vi "SpectrometerSpinCoater_v08.vi"() -> ()   [LabVIEW 2018]
uses:
  <instrlib>/Classes/CCD/Abstract_CCD/Abstract_CCD.lvclass
  <instrlib>/Classes/SpinCoater/SpinCoater.lvclass
  TypDef/DeviceQueue_TypeDef.ctl
  TypDef/DeviceQueue_Action.ctl
  TypDef/TabControl.ctl
  TypDef/DataQueue_TypeDef.ctl
  TypDef/DataQueue_Action.ctl
  <vilib>/Utility/error.llb/DialogType.ctl
  <instrlib>/Classes/CCD/Avantes/Avantes.lvclass
  C:/Program Files/National Instruments/LabVIEW 2018/instr.lib/Classes/CCD/Abstract_CCD/Abstract_CCD.lvclass
  <vilib>/Analysis/baseanly.llb/A x Vector.vi
  <vilib>/Analysis/NI_AALBase.lvlib
panel:
  out "Nr After Spin":u16=6
  out "Action":string="TimeOut"
  out "Time.spin":refnum<file>
  out "Meas.spin":refnum<file>
  out "Arduino":bool
  out "NKT":bool
  out "Spectromter":bool
  in  "Abort Button":bool
  in  "Stop Button":bool=TRUE
  in  "Tab Control":T1(tab)
  in  "Spin at end":bool=TRUE
  in  "Duration after":dbl[unit]=10.0
  in  "periodic time":dbl[unit]=2.0
  in  "Program Spin Coater":T2(array[cluster])=[{"Speed (rpm)"=1500.0, "Time (s)"=5.0, "Acc (rpm/s)"=0.0}]
  in  "Spectra Count":u16
  in  "Measure_MeasureSpectrum":bool
  out "Overall Time":dbl=6.5
  in  "Seconds after Spin":dbl[unit]=0.5
  in  "Seconds to Spin":dbl[unit]=1.0
  in  "Calculate Frames":bool=TRUE
  in  "Frames":i32=17106
  in  "StartMeasurement_Button":bool
  in  "Measure_Preview":bool
  out "Measure_Graph":T3(graph) caption="XY Graph"
  in  "Measure_FramesSpectrometer":dbl=200.0 caption="Frames for Spectrometer"
  in  "StartSpin_Button":bool
  in  "Record RefSpec":bool
  in  "Record_Darkspec":bool
  in  "Measure_Comments":string="Just for testing" caption="Comments"
  in  "Measure_FileName":string="TestingAfter" caption="File Name"
  in  "Measure_SavePath":path=path "C:/Users/Timo/Desktop/Test/180824" caption="Save Path"
  out "Measure_FrameRate":dbl[unit]=2631.5791015625 caption="Frame Rate"
  in  "Measure_IntegrationTime":dbl[unit]=3e-05 caption="Integration Time"
  in  "Dividider Get Spectra":u32=1 min=1
  in  "Automatically \nadjust count":bool=TRUE
  in  "Reset Count\nafter Spin Coating":bool=TRUE
  in  "Speed":dbl
  in  "Milliseconds":dbl
  in  "Debug":bool
  in  "Port Arduino":refnum<visa-resource-name>="COM3"
  out "Error Arduino":bool caption="Error"
  in  "Init_Arduino":bool=TRUE caption="Init"
  out "Caption_Settings_Arduino":string="Arduino"
  out "Caption_Settings_NKT":string="NKT Laser"
  out "Error_Spectromter":bool caption="Error"
  in  "Init_Spectrometer":bool=TRUE caption="Init"
  out "Caption_Settings_Spectrometer":string="Spectromter"
  # "Speed (rpm)   Time (s)        Acceleration \n                                               (rpm/s)"
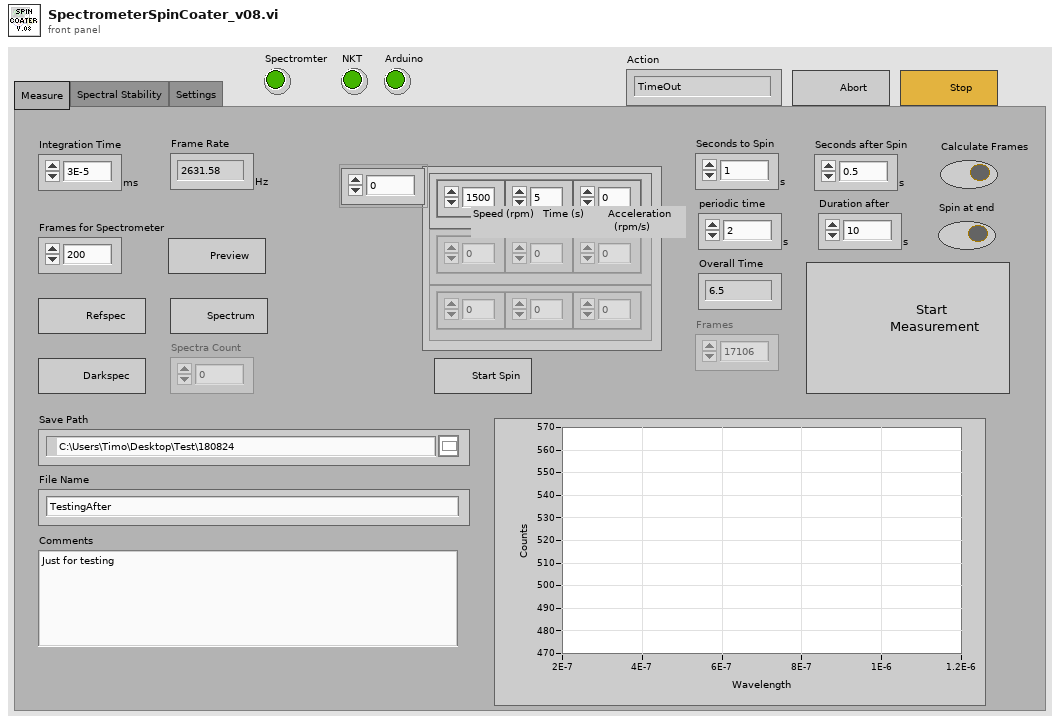
[diagram p1: front panel]
types:
  T1 = enum32{"Measure", "Spectral Stability", "Settings"}
  T2 = cluster{"Speed (rpm)":dbl, "Time (s)":dbl, "Acc (rpm/s)":dbl}[]
  T3 = cluster{"Wavlength":dbl[unit][], "Image":dbl[]}[]
  T4 = cluster{"Dark":cluster{"Image":dbl[][][], "Frame Size":cluster{"F":i32, "Y":i32, "X":i32}}[], "Ref":cluster{"Image":dbl[][][], "Frame Size":cluster{"F":i32, "Y":i32, "X":i32}}[], "Wavlength":dbl[unit][], "spec":dbl[][]}
  T5 = cluster{"Abstract_CCD.lvclass":refnum<class "Abstract_CCD.lvclass">, "SpinCoater.lvclass":refnum<class "SpinCoater.lvclass">}
  T6 = typedef "DataQueue_TypeDef.ctl" = cluster{"QueueAction":T7, "Data":cluster{"Image":dbl[][][], "Frame Size":cluster{"F":i32, "Y":i32, "X":i32}}[], "Data_Raw":cluster{"Image":dbl[][][], "Frame Size":cluster{"F":i32, "Y":i32, "X":i32}}[], "Data_Dark":cluster{"Image":dbl[][][], "Frame Size":cluster{"F":i32, "Y":i32, "X":i32}}[], "Data_Ref":cluster{"Image":dbl[][][], "Frame Size":cluster{"F":i32, "Y":i32, "X":i32}}[], "Device Information":string[], "Numeric Control":dbl, "Boolean":bool, "Wavelength":dbl[unit][], "Time":dbl[], "Time Stamp":timestamp, "Numeric Control 2":dbl, "TabControl":T8}
  T7 = typedef "DataQueue_Action.ctl" = enum16{"TimeOut", "Close_Program", "Stop_Measurement", "Measure_InSituSpinCoating", "Measure_Spectrum", "Measure_SpectrumAdvanced", "Save_InSitu", "Save_SpectralStability", "Set_Ref", "Set_Dark", "Set_Wavelength", "Spectrometer_Measure", "Spectrometer_Preview", "Transfer_Settings"}
  T8 = typedef "TabControl.ctl" = enum16{"Measure", "Spectral Stability", "Settings"}
  T9 = typedef "DeviceQueue_TypeDef.ctl" = cluster{"QueueAction":T10, "Numeric 1":dbl, "Numeric 2":dbl, "Boolean 1":bool, "Boolean 2":bool, "Spin Program":dbl[][], "Spin Prg v07":cluster{"Speed (rpm)":dbl, "Time (s)":dbl, "Acc (rpm/s)":dbl}[], "Time Stamp":timestamp, "TabControl":T8}
  T10 = typedef "DeviceQueue_Action.ctl" = enum16{"TimeOut", "Wait", "Close_Program", "Abort", "Spectrometer_Init", "Spectrometer_Close", "Spectrometer_DeviceInformation", "Spectrometer_Measure", "Spectrometer_MeasureAdvanced", "Spectrometer_Preview", "Spectrometer_Abort", "Spectrometer_StartMeasurement", "Spectrometer_GetData", "Spectrometer_StopMeasurement", "Spectrometer_SetIntegrationTime", "Spectrometer_SetFrames", "Spectrometer_SetDarkspec", "Spectrometer_SetReference", "Spectrometer_SetTriggerMode", "Laser_Init", "Laser_Close", "Arduino_Init", "Arduino_Close", "Arduino_LoadProgram", "Arduino_StartProgram", "Arduino_SetSpeed", "Arduino_SetMillis", "Arduino_StopSpin", "Measure_InSitu", "Measure_Spectrum", "Measure_InSituAdvanced", "Measure_Stop"}
  T11 = enum16{"open", "replace", "create", "open or create", "replace or create", "replace or create with confirmation"}
  T12 = cluster{"Image":dbl[][][], "Frame Size":cluster{"F":i32, "Y":i32, "X":i32}}[]
  T13 = cluster{"Image":dbl[][][], "Frame Size":cluster{"F":i32, "Y":i32, "X":i32}}
  T14 = cluster{"Wavlength":dbl[unit][], "A x Vector":dbl[]}
  T15 = cluster{"Wavlength":dbl[unit][], "A x Vector":dbl[]}[]
  T16 = cluster{u16[][], u16[][], dbl[], "Numeric Control":dbl, "Numeric Control 2":dbl}
  T17 = typedef "DialogType.ctl" = u16
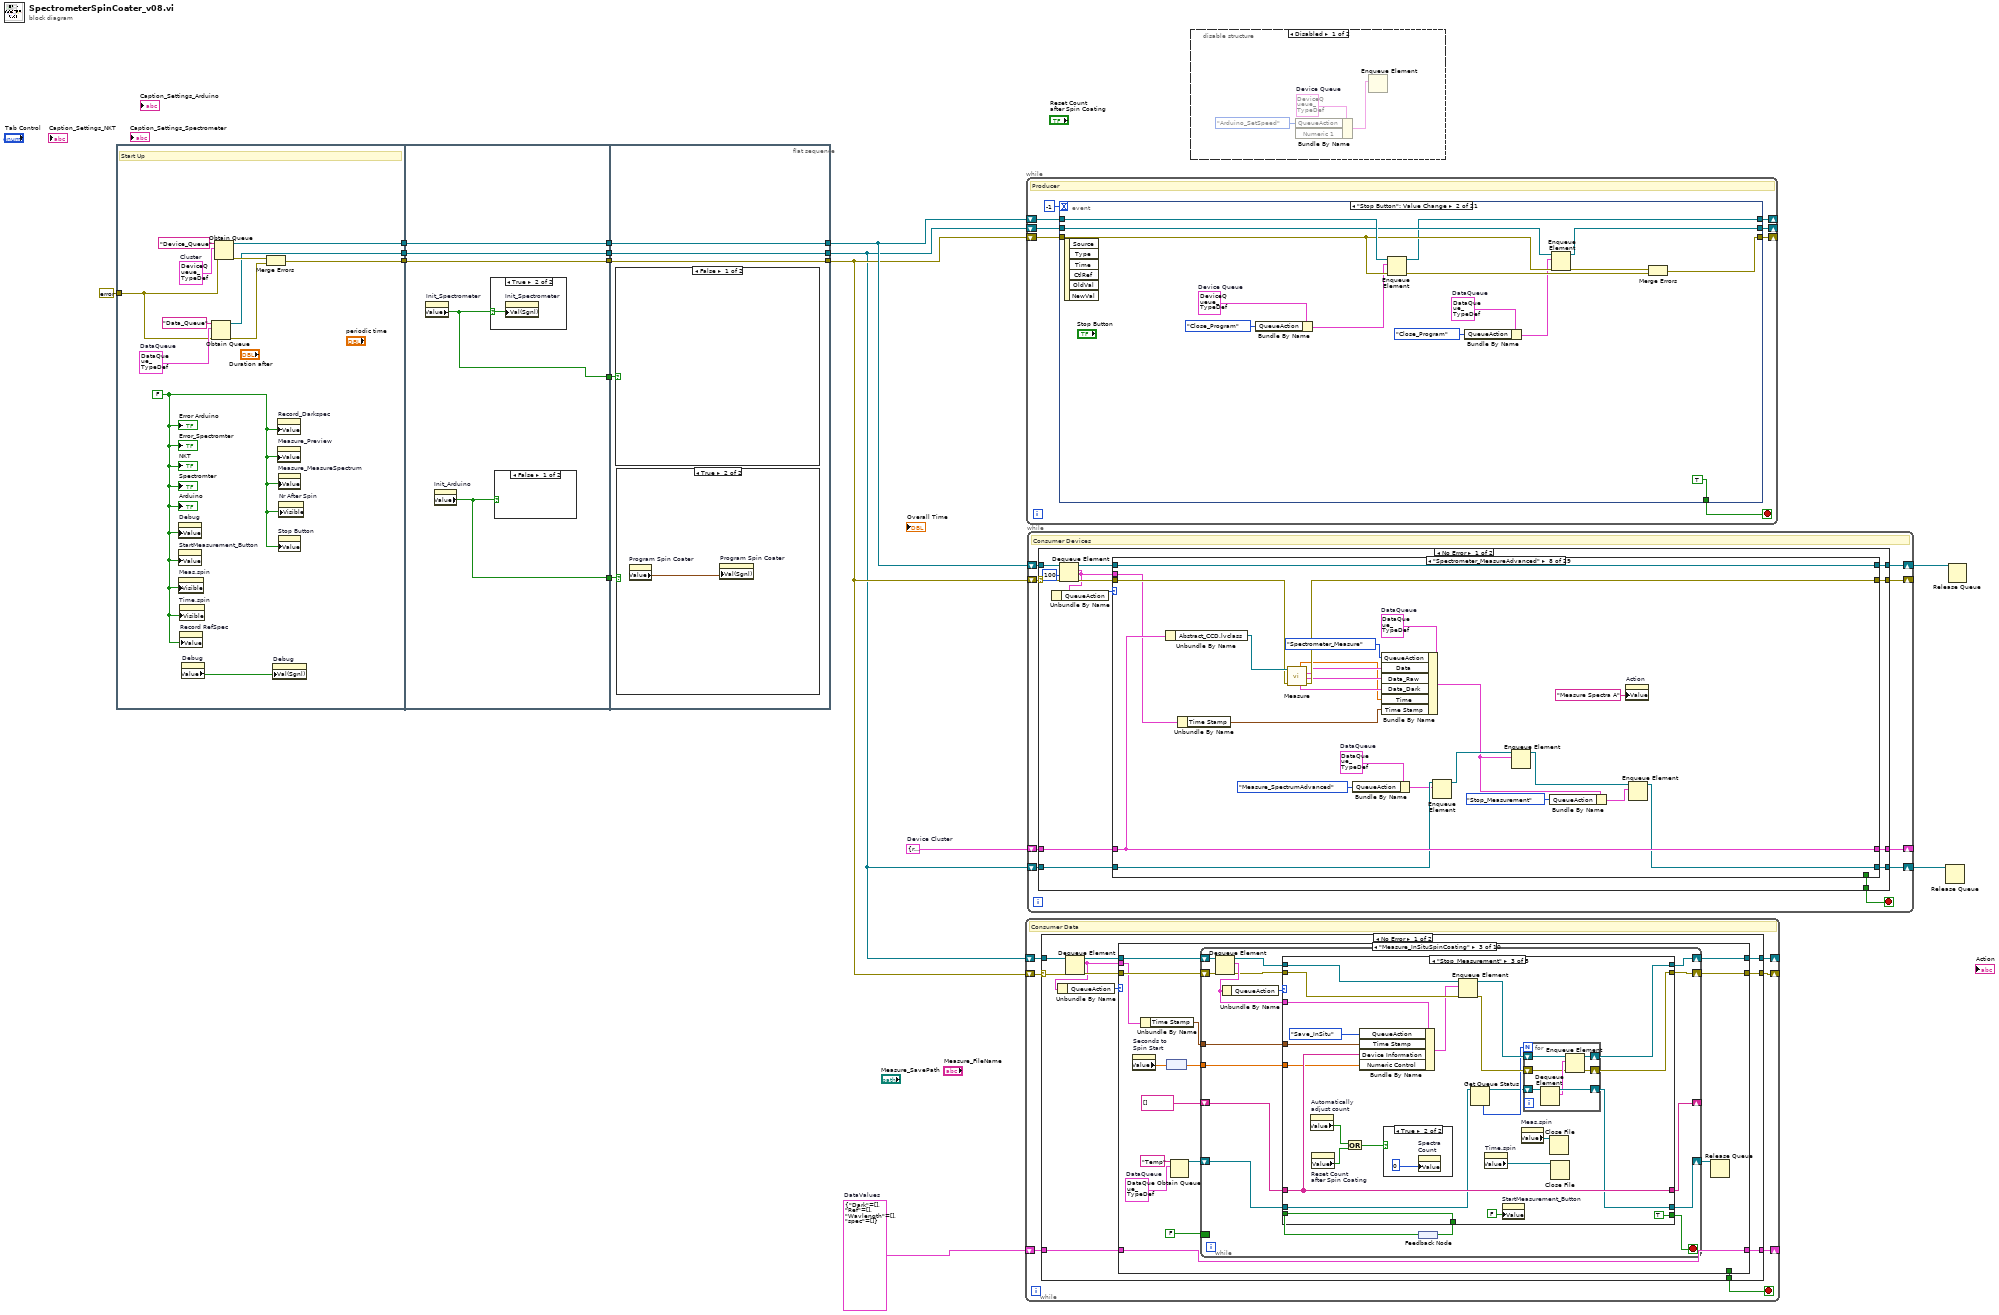
[diagram p0: block diagram]
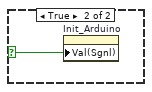
[diagram p3: hidden frame]
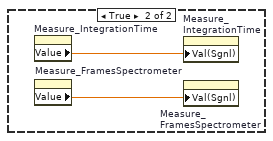
[diagram p6: hidden frame]
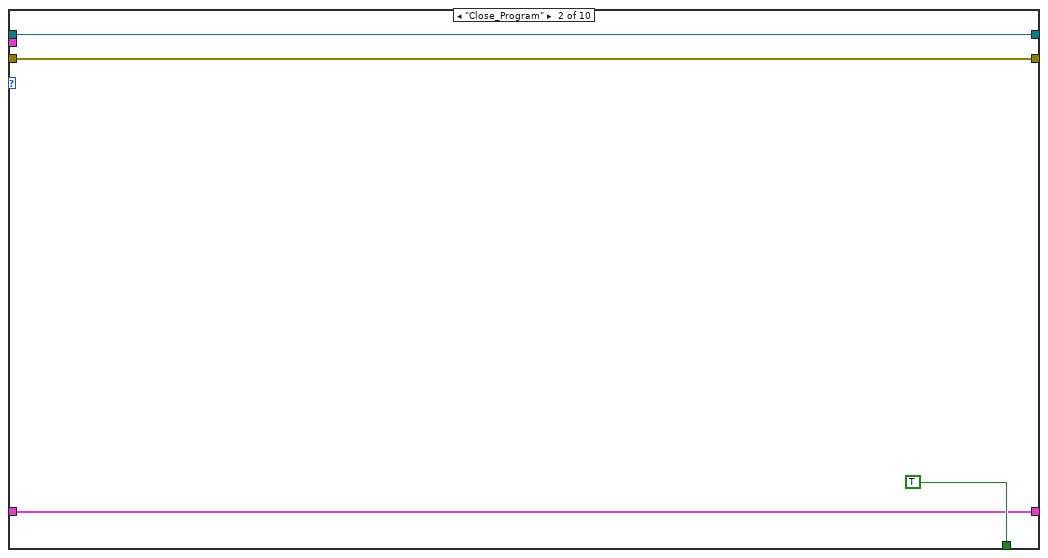
[diagram p8: hidden frame]
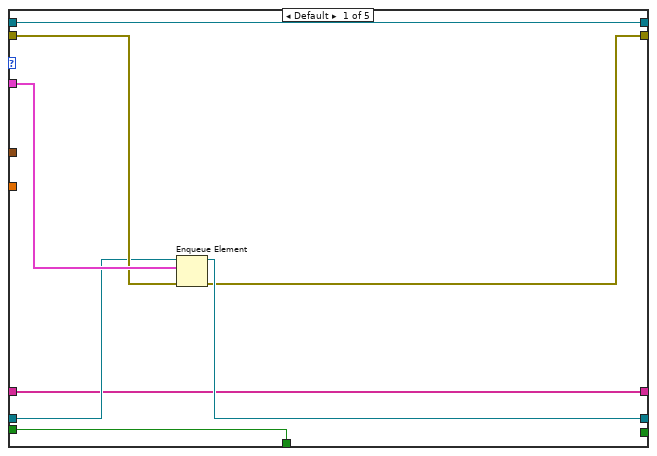
[diagram p9: hidden frame]
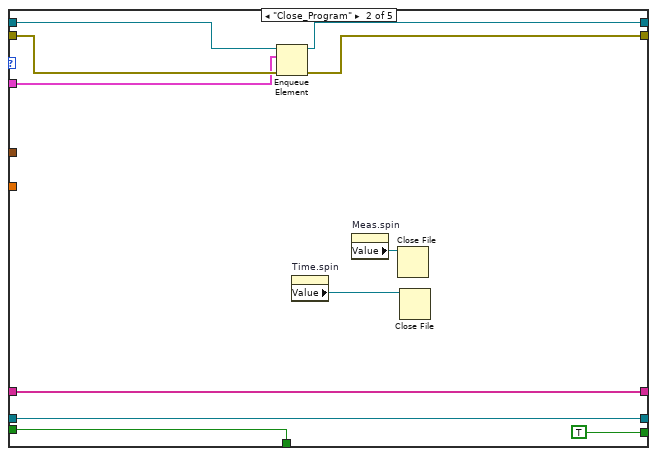
[diagram p10: hidden frame]
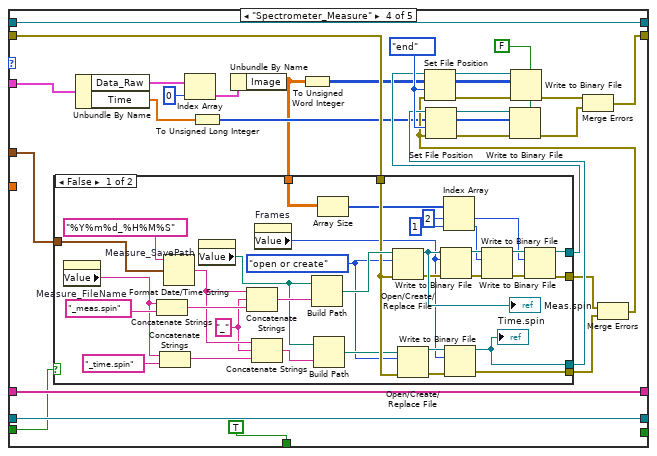
[diagram p12: hidden frame]
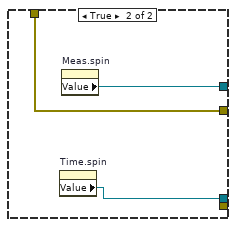
[diagram p13: hidden frame]
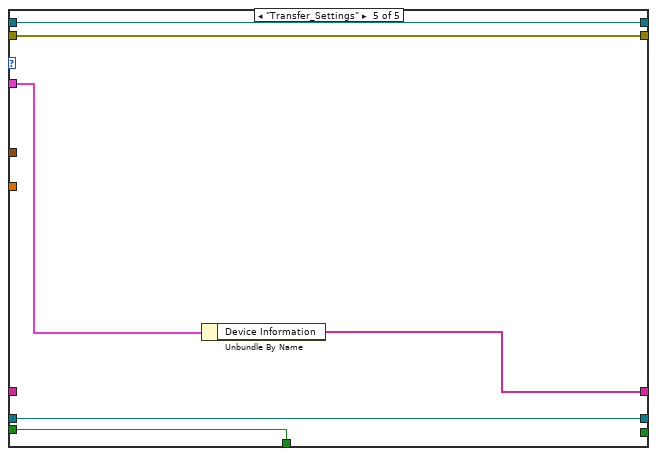
[diagram p14: hidden frame]
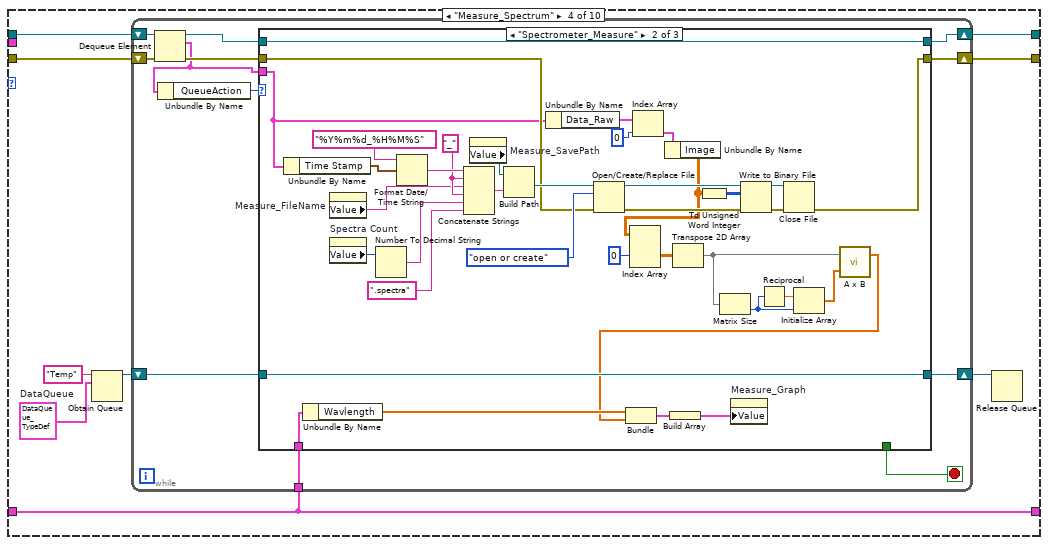
[diagram p15: hidden frame]
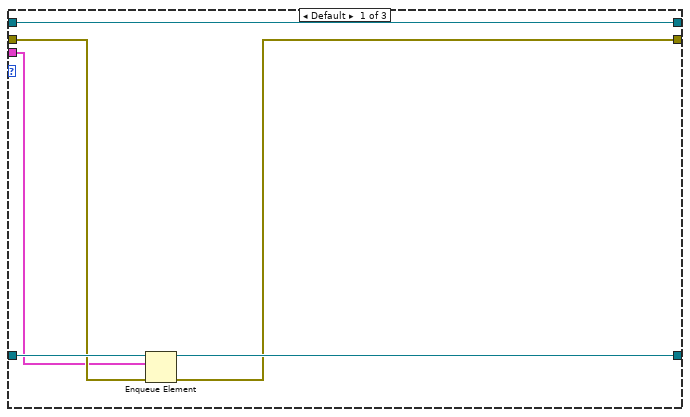
[diagram p16: hidden frame]
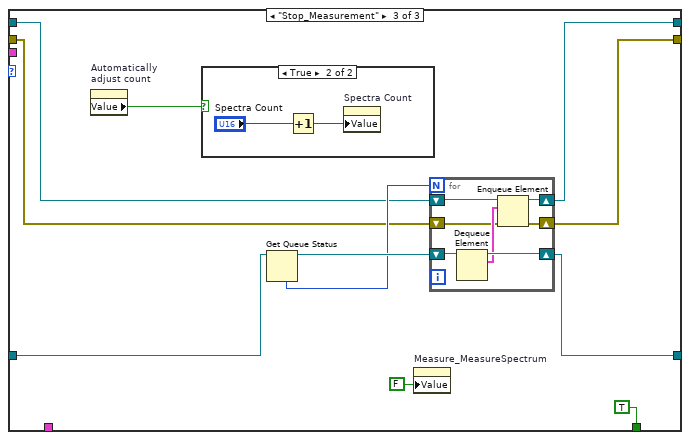
[diagram p17: hidden frame]
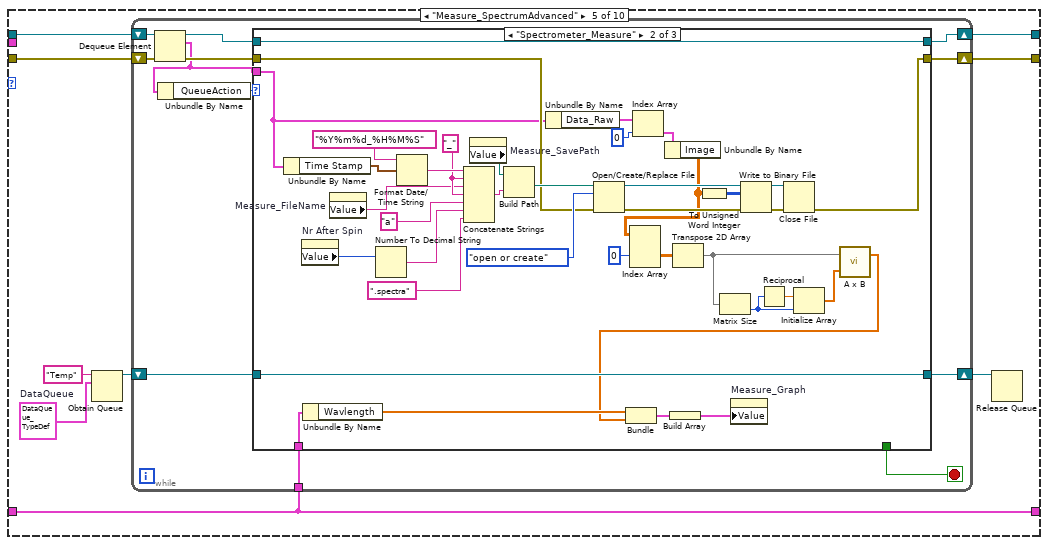
[diagram p19: hidden frame]
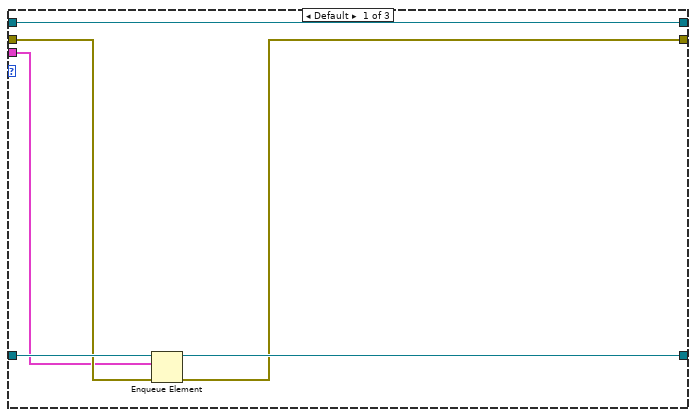
[diagram p20: hidden frame]
diagram:
  w6 = T4 {"Dark"=[], "Ref"=[], "Wavlength"=[], "spec"=[]}  # DataValues
  w11 = T5 {"Abstract_CCD.lvclass"=refnum, "SpinCoater.lvclass"=refnum}  # Device Cluster
  n1 = flat-sequence {
    tunnel: errorcluster {"status"=FALSE, "code"=0, "source"=""} ("error constant") -> [w23]
    tunnel: [w26] -> w15
    tunnel: [w20] -> w14
    tunnel: [w19] -> w13
    tunnel: w15 -> [w33]
    tunnel: w14 -> [w32]
    tunnel: w13 -> [w31]
    tunnel: [w33] -> w5
    tunnel: [w32] -> w4
    tunnel: [w31] -> w3
    tunnel: [w30] -> w2
    tunnel: [w29] -> w1
    tunnel: [w38] -> w8
    tunnel: [w39] -> w7
    tunnel: [w40] -> w12
    tunnel: w5 -> [w40]
    tunnel: w4 -> [w39]
    tunnel: w3 -> [w38]
    tunnel: w2 -> [w37]
    tunnel: w1 -> [w36]
    frame #0 {
      w24 = T6 {"QueueAction"=enum."TimeOut", "Data"=[], "Data_Raw"=[], "Data_Dark"=[], "Data_Ref"=[], "Device Information"=[], "Numeric Control"=0.0, "Boolean"=FALSE, "Wavelength"=[], "Time"=[], "Time Stamp"=timestamp(0 s since 1904-01-01), "Numeric Control 2"=0.0, "TabControl"=enum."Measure"}  # DataQueue
      w27 = T9 {"QueueAction"=enum."TimeOut", "Numeric 1"=0.0, "Numeric 2"=0.0, "Boolean 1"=FALSE, "Boolean 2"=FALSE, "Spin Program"=[], "Spin Prg v07"=[], "Time Stamp"=timestamp(0 s since 1904-01-01), "TabControl"=enum."Measure"}  # Cluster
      w17 = FALSE ("Error Arduino")
      # "Start Up"
      n2 = property on="Debug" class="Bool (strict)"("Value"=w17) -> ()  [unwired: 2 in, 2 out]
      n3 = property on="StartMeasurement_Button" class="Bool (strict)"("Value"=w17) -> ()  [unwired: 2 in, 2 out]
      n4 = property on="Meas.spin" class="Ref (strict)"("Visible"=w17) -> ()  [unwired: 2 in, 2 out]
      n5 = property on="Time.spin" class="Ref (strict)"("Visible"=w17) -> ()  [unwired: 2 in, 2 out]
      n6 = property on="Record RefSpec" class="Bool (strict)"("Value"=w17) -> ()  [unwired: 2 in, 2 out]
      n7 = property on="Debug" class="Bool (strict)"() -> ("Value"=w18:bool)  [unwired: 2 in, 2 out]
      n8 = Obtain Queue(name (unnamed)="Data_Queue", element data type=w24, error in (no error)=w23) -> (queue out=w20:refnum<queue>, error out=w21:errorcluster)  [unwired: 2 in, 1 out]
      n9 = Obtain Queue(name (unnamed)="Device_Queue", element data type=w27, error in (no error)=w23) -> (queue out=w26:refnum<queue>, error out=w22:errorcluster)  [unwired: 2 in, 1 out]
      n10 = Merge Errors(w22, w21) -> (w19:errorcluster)
      n11 = property on="Debug" class="Bool (strict)"("Val(Sgnl)"=w18) -> ()  [unwired: 2 in, 2 out]
      n12 = property on="Record_Darkspec" class="Bool (strict)"("Value"=w17) -> ()  [unwired: 2 in, 2 out]
      n13 = property on="Measure_Preview" class="Bool (strict)"("Value"=w17) -> ()  [unwired: 2 in, 2 out]
      n14 = property on="Measure_MeasureSpectrum" class="Bool (strict)"("Value"=w17) -> ()  [unwired: 2 in, 2 out]
      n15 = property on="Stop Button" class="Bool (strict)"("Value"=w17) -> ()  [unwired: 2 in, 2 out]
      n16 = property on="Nr After Spin" class="DigNum (strict)"("Visible"=w17) -> ()  [unwired: 2 in, 2 out]
      "Error_Spectromter" <- w17
      "Error Arduino" <- w17
      "Spectromter" <- w17
      "NKT" <- w17
      "Arduino" <- w17
    }
    frame #1 {
      n17 = property on="Init_Spectrometer" class="Bool (strict)"() -> ("Value"=w30:bool)  [unwired: 2 in, 2 out]
      n18 = property on="Init_Arduino" class="Bool (strict)"() -> ("Value"=w29:bool)  [unwired: 2 in, 2 out]
      n19 = case shown="True" w30 {
        selector: w30 -> [_ w35]
        frame False {
        }
        frame True {
          n20 = property on="Init_Spectrometer" class="Bool (strict)"("Val(Sgnl)"=w35) -> ()  [unwired: 2 in, 2 out]
        }
      }
      n21 = case shown="False" w29 {
        selector: w29 -> [_ w34]
        frame False {
        }
        frame True {
          n22 = property on="Init_Arduino" class="Bool (strict)"("Val(Sgnl)"=w34) -> ()  [unwired: 2 in, 2 out]
        }
      }
    }
    frame #2 {
      n23 = case shown="False" w37 {
        frame False {
        }
        frame True {
          n24 = property on="Measure_IntegrationTime" class="DigNum (strict)"() -> ("Value"=w42:dbl[unit])  [unwired: 2 in, 2 out]
          n25 = property on="Measure_FramesSpectrometer" class="DigNum (strict)"() -> ("Value"=w43:dbl)  [unwired: 2 in, 2 out]
          n26 = property on="Measure_IntegrationTime" class="DigNum (strict)"("Val(Sgnl)"=w42) -> ()  [unwired: 2 in, 2 out]
          n27 = property on="Measure_FramesSpectrometer" class="DigNum (strict)"("Val(Sgnl)"=w43) -> ()  [unwired: 2 in, 2 out]
        }
      }
      n28 = case shown="True" w36 {
        frame False {
        }
        frame True {
          n29 = property on="Program Spin Coater" class="Arr (strict)"() -> ("Value"=w41:T2)  [unwired: 2 in, 2 out]
          n30 = property on="Program Spin Coater" class="Arr (strict)"("Val(Sgnl)"=w41) -> ()  [unwired: 2 in, 2 out]
        }
      }
    }
  }
  n31 = while {
    shift-right: [w44] -> _
    shift-left: w8 -> [w50]
    shift-right: [w45] -> _
    shift-left: w7 -> [w49]
    shift-right: [w46] -> _
    shift-left: w6 -> [w48]
    stop <- w47 stop-if-true
    # "Consumer Data"
    n32 = case shown="No Error" w50 {
      selector: w50 -> [w61 w509]
      tunnel: w49 -> [w60 w510]
      tunnel: w48 -> [w58 w507]
      tunnel: [w57 _] -> w47
      tunnel: [w56 w507] -> w46
      tunnel: [w55 w510] -> w45
      tunnel: [w53 w508] -> w44
      frame No Error {
        n33 = Dequeue Element(queue=w60, error in (no error)=w61) -> (queue out=w54:refnum<queue>, element=w51:T6, error out=w52:errorcluster)  [unwired: 1 in, 1 out]
        n34 = Unbundle By Name(w51) -> ("QueueAction"=w59:T7)
        n35 = case shown="\"Measure_InSituSpinCoating\"" w59 {
          tunnel: w58 -> [w62 w67 w73 w225 w309 w421 w461 w470 w492 w503]
          tunnel: [_ TRUE _ _ _ _ _ _ _ _] -> w57
          tunnel: [w62 w67 w73 w225 w309 w421 w465 w484 w491 w503] -> w56
          tunnel: [w64 w66 w83 w231 w315 w448 w466 w485 w488 w506] -> w55
          tunnel: w54 -> [w64 w66 w81 w232 w316 w448 w466 w485 w488 w506]
          tunnel: [w63 w65 w82 w230 w314 w447 w467 w486 w489 w505] -> w53
          tunnel: w52 -> [w63 w65 w80 w233 w317 w447 w467 w486 w489 w505]
          tunnel: w51 -> [_ _ w75 _ _ w434 w468 w487 w490 w504]
          frame "TimeOut", Default {
          }
          frame "Close_Program" {
          }
          frame "Measure_InSituSpinCoating" {
            w78 = T6 {"QueueAction"=enum."TimeOut", "Data"=[], "Data_Raw"=[], "Data_Dark"=[], "Data_Ref"=[], "Device Information"=[], "Numeric Control"=0.0, "Boolean"=FALSE, "Wavelength"=[], "Time"=[], "Time Stamp"=timestamp(0 s since 1904-01-01), "Numeric Control 2"=0.0, "TabControl"=enum."Measure"}  # DataQueue
            n36 = property on="Seconds to\nSpin Start" class="DigNum (strict)"() -> ("Value"=w70:dbl[unit])  [unwired: 2 in, 2 out]
            n37 = Unbundle By Name(w75) -> ("Time Stamp"=w74:timestamp)
            n38 = node(w70) -> (w69:dbl)
            n39 = Obtain Queue(name (unnamed)="Temp", element data type=w78) -> (queue out=w77:refnum<queue>)  [unwired: 3 in, 2 out]
            n40 = while {
              shift-right: [w91] -> w83
              shift-left: w81 -> [w100]
              shift-right: [w92] -> w82
              shift-left: w80 -> [w99]
              shift-right: [w93] -> w76
              shift-left: w77 -> [w94]
              tunnel: w74 -> [w87]
              shift-right: [w88] -> _
              shift-left: string[] [] ("Device Information") -> [w89]
              border: FALSE -> [_]
              tunnel: w69 -> [w84]
              stop <- w90 stop-if-true
              n41 = Dequeue Element(queue=w100, error in (no error)=w99) -> (queue out=w95:refnum<queue>, element=w97:T6, error out=w96:errorcluster)  [unwired: 1 in, 1 out]
              n42 = Unbundle By Name(w97) -> ("QueueAction"=w98:T7)
              n43 = feedback #1() -> (w86:bool)
              n44 = case shown="\"Stop_Measurement\"" w98 {
                tunnel: w97 -> [w108 w117 w142 w179 w223]
                tunnel: w96 -> [w107 w118 w139 w170 w220]
                tunnel: w95 -> [w103 w119 w138 w178 w221]
                tunnel: w94 -> [w106 w114 w133 w167 w224]
                tunnel: [w105 w114 w130 w167 w224] -> w93
                tunnel: [w104 w115 w129 w168 w220] -> w92
                tunnel: [w103 w116 w128 w178 w221] -> w91
                tunnel: [_ TRUE TRUE _ _] -> w90
                tunnel: w89 -> [w102 w112 w140 w165 _]
                tunnel: [w102 w112 w140 w165 w222] -> w88
                tunnel: w87 -> [_ _ w141 w180 _]
                tunnel: w86 -> [w101 w111 w127 w163 w219]
                tunnel: [w101 w111 w127 TRUE w219] -> w85
                tunnel: w84 -> [_ _ w124 _ _]
                frame Default {
                  n45 = Enqueue Element(queue=w106, element=w108, error in (no error)=w107) -> (queue out=w105:refnum<queue>, error out=w104:errorcluster)  [unwired: 1 in, 1 out]
                }
                frame "Close_Program" {
                  n46 = Enqueue Element(queue=w119, element=w117, error in (no error)=w118) -> (queue out=w116:refnum<queue>, error out=w115:errorcluster)  [unwired: 1 in, 1 out]
                  n47 = property on="Time.spin" class="Ref (strict)"() -> ("Value"=w109:refnum<file>)  [unwired: 2 in, 2 out]
                  n48 = property on="Meas.spin" class="Ref (strict)"() -> ("Value"=w110:refnum<file>)  [unwired: 2 in, 2 out]
                  n49 = Close File(refnum=w110) -> ()  [unwired: 1 in, 2 out]
                  n50 = Close File(refnum=w109) -> ()  [unwired: 1 in, 2 out]
                }
                frame "Stop_Measurement" {
                  n51 = property on="Automatically \nadjust count" class="Bool (strict)"() -> ("Value"=w121:bool)  [unwired: 2 in, 2 out]
                  n52 = property on="Reset Count\nafter Spin Coating" class="Bool (strict)"() -> ("Value"=w122:bool)  [unwired: 2 in, 2 out]
                  n53 = Or(x=w121, y=w122) -> (x .or. y?=w120:bool)
                  n54 = Bundle By Name(cluster=w142, "QueueAction"=DataQueue_Action."Save_InSitu", "Time Stamp"=w141, "Device Information"=w140, "Numeric Control"=w124) -> (w137:T6)
                  n55 = case shown="True" w120 {
                    frame False {
                    }
                    frame True {
                      n56 = property on="Spectra \nCount" class="DigNum (strict)"("Value"=u16 0 ("Spectra Count")) -> ()  [unwired: 2 in, 2 out]
                    }
                  }
                  n57 = Enqueue Element(queue=w138, element=w137, error in (no error)=w139) -> (queue out=w135:refnum<queue>, error out=w134:errorcluster)  [unwired: 1 in, 1 out]
                  n58 = Get Queue Status(queue=w133) -> (queue out=w131:refnum<queue>, # elements in queue=w132:i32)  [unwired: 2 in, 6 out]
                  n59 = property on="Time.spin" class="Ref (strict)"() -> ("Value"=w125:refnum<file>)  [unwired: 2 in, 2 out]
                  n60 = property on="StartMeasurement_Button" class="Bool (strict)"("Value"=FALSE ("StartMeasurement_Button")) -> ()  [unwired: 2 in, 2 out]
                  n61 = property on="Meas.spin" class="Ref (strict)"() -> ("Value"=w126:refnum<file>)  [unwired: 2 in, 2 out]
                  n62 = for {
                    N: w132 -> [_]
                    shift-right: [w150] -> w130
                    shift-left: w131 -> [w151]
                    shift-right: [w147] -> w128
                    shift-left: w135 -> [w148]
                    shift-right: [w145] -> w129
                    shift-left: w134 -> [w146]
                    n63 = Dequeue Element(queue=w151) -> (queue out=w150:refnum<queue>, element=w149:T6)  [unwired: 2 in, 2 out]
                    n64 = Enqueue Element(queue=w148, element=w149, error in (no error)=w146) -> (queue out=w147:refnum<queue>, error out=w145:errorcluster)  [unwired: 1 in, 1 out]
                  }
                  n65 = Close File(refnum=w126) -> ()  [unwired: 1 in, 2 out]
                  n66 = Close File(refnum=w125) -> ()  [unwired: 1 in, 2 out]
                }
                frame "Spectrometer_Measure" {
                  w153 = FALSE ("prepend array or string size? (T)")
                  w166 = enum16{"start", "end", "current"}."end" ("from (0:start)")
                  n67 = Unbundle By Name(w179) -> ("Data_Raw"=w175:T12, "Time"=w169:dbl[])
                  n68 = Index Array(array=w175, index=0) -> (element=w174:T13)
                  n69 = To Unsigned Long Integer(number=w169) -> (unsigned 32bit integer=w155:u32[])
                  n70 = Unbundle By Name(w174) -> ("Image"=w152:dbl[][][])
                  n71 = case shown="False" w163 {
                    tunnel: w180 -> [w212 _]
                    tunnel: w170 -> [w207 w218]
                    tunnel: [w193 w218] -> w157
                    tunnel: [w181 _] -> w158
                    tunnel: [w192 w217] -> w160
                    tunnel: [w182 w216] -> w159
                    tunnel: w152 -> [w190 _]
                    frame False {
                      w202 = T11."open or create" ("operation (0:open)")
                      w201 = "_" ("string")
                      n72 = property on="Measure_FileName" class="Str"() -> ("Value"=w210:string)  [unwired: 2 in, 2 out]
                      n73 = Concatenate Strings(w210, "_meas.spin" ("string")) -> (w213:string)
                      n74 = Concatenate Strings(w210, "_time.spin" ("string")) -> (w205:string)
                      n75 = Format Date/Time String(time format string (%c)="%Y%m%d_%H%M%S", seconds (now)=w212) -> (date/time string=w206:string)  [unwired: 1 in]
                      n76 = property on="Measure_SavePath" class="Path"() -> ("Value"=w184:path)  [unwired: 2 in, 2 out]
                      n77 = Concatenate Strings(w206, w201, w213) -> (w211:string)
                      n78 = Concatenate Strings(w206, w201, w205) -> (w204:string)
                      n79 = property on="Frames" class="DigNum (strict)"() -> ("Value"=w183:i32)  [unwired: 2 in, 2 out]
                      n80 = Build Path(base path=w184, name or relative path=w211) -> (appended path=w208:path)
                      n81 = Build Path(base path=w184, name or relative path=w204) -> (appended path=w203:path)
                      n82 = Array Size(array=w190) -> (size(s)=w189:i32[])
                      n83 = Open/Create/Replace File(file path (use dialog)=w208, error in=w207, operation (0:open)=w202) -> (refnum out=w200:refnum<file>, error out=w199:errorcluster)  [unwired: 3 in, 1 out]
                      "Meas.spin" <- w200
                      n84 = Open/Create/Replace File(file path (use dialog)=w203, error in=w207, operation (0:open)=w202) -> (refnum out=w198:refnum<file>, error out=w197:errorcluster)  [unwired: 3 in, 1 out]
                      n85 = Write to Binary File(file (use dialog)=w200, data=w183, error in=w199) -> (refnum out=w196:refnum<file>, error out=w195:errorcluster)  [unwired: 3 in, 1 out]
                      n86 = Index Array(array=w189, index #1=2 ("index"), index #2=1 ("index")) -> (element #1=w185:i32, element #2=w186:i32)
                      n87 = Write to Binary File(file (use dialog)=w198, data=w183, error in=w197) -> (refnum out=w182:refnum<file>, error out=w181:errorcluster)  [unwired: 3 in, 1 out]
                      "Time.spin" <- w182
                      n88 = Write to Binary File(file (use dialog)=w196, data=w186, error in=w195) -> (refnum out=w191:refnum<file>, error out=w194:errorcluster)  [unwired: 3 in, 1 out]
                      n89 = Write to Binary File(file (use dialog)=w191, data=w185, error in=w194) -> (refnum out=w192:refnum<file>, error out=w193:errorcluster)  [unwired: 3 in, 1 out]
                    }
                    frame True {
                      n90 = property on="Time.spin" class="Ref (strict)"() -> ("Value"=w216:refnum<file>)  [unwired: 2 in, 2 out]
                      n91 = property on="Meas.spin" class="Ref (strict)"() -> ("Value"=w217:refnum<file>)  [unwired: 2 in, 2 out]
                    }
                  }
                  n92 = To Unsigned Word Integer(number=w152) -> (unsigned 16bit integer=w154:u16[][][])
                  n93 = Merge Errors(w157, w158) -> (w156:errorcluster)
                  n94 = Set File Position(refnum=w160, from (0:start)=w166, error in=w156) -> (refnum out=w172:refnum<file>, error out=w171:errorcluster)  [unwired: 1 in]
                  n95 = Set File Position(refnum=w159, from (0:start)=w166, error in=w156) -> (refnum out=w177:refnum<file>, error out=w176:errorcluster)  [unwired: 1 in]
                  n96 = Write to Binary File(file (use dialog)=w177, data=w155, error in=w176, 5:w153) -> (error out=w161:errorcluster)  [unwired: 2 in, 2 out]
                  n97 = Write to Binary File(file (use dialog)=w172, data=w154, error in=w171, 5:w153) -> (error out=w162:errorcluster)  [unwired: 2 in, 2 out]
                  n98 = Merge Errors(w162, w161) -> (w168:errorcluster)
                }
                frame "Transfer_Settings" {
                  n99 = Unbundle By Name(w223) -> ("Device Information"=w222:string[])
                }
              }
              n100 = feedback-in #1(w85) -> ()
            }
            n101 = Release Queue(queue=w76) -> ()  [unwired: 2 in, 3 out]
          }
          frame "Measure_Spectrum" {
            w228 = T6 {"QueueAction"=enum."TimeOut", "Data"=[], "Data_Raw"=[], "Data_Dark"=[], "Data_Ref"=[], "Device Information"=[], "Numeric Control"=0.0, "Boolean"=FALSE, "Wavelength"=[], "Time"=[], "Time Stamp"=timestamp(0 s since 1904-01-01), "Numeric Control 2"=0.0, "TabControl"=enum."Measure"}  # DataQueue
            n102 = Obtain Queue(name (unnamed)="Temp", element data type=w228) -> (queue out=w227:refnum<queue>)  [unwired: 3 in, 2 out]
            n103 = while {
              shift-right: [w236] -> w231
              shift-left: w232 -> [w244]
              shift-right: [w237] -> w230
              shift-left: w233 -> [w245]
              shift-right: [w238] -> w226
              shift-left: w227 -> [w240]
              tunnel: w225 -> [w234]
              stop <- w235 stop-if-true
              n104 = Dequeue Element(queue=w244, error in (no error)=w245) -> (queue out=w242:refnum<queue>, element=w239:T6, error out=w241:errorcluster)  [unwired: 1 in, 1 out]
              n105 = Unbundle By Name(w239) -> ("QueueAction"=w243:T7)
              n106 = case shown="\"Spectrometer_Measure\"" w243 {
                tunnel: w242 -> [w246 w266 w295]
                tunnel: w241 -> [w249 w276 w294]
                tunnel: w240 -> [w251 w287 w297]
                tunnel: w239 -> [w247 w253 _]
                tunnel: [w250 w287 w293] -> w238
                tunnel: [w248 w267 w291] -> w237
                tunnel: [w246 w266 w292] -> w236
                tunnel: [_ _ TRUE] -> w235
                tunnel: w234 -> [_ w258 _]
                frame Default {
                  n107 = Enqueue Element(queue=w251, element=w247, error in (no error)=w249) -> (queue out=w250:refnum<queue>, error out=w248:errorcluster)  [unwired: 1 in, 1 out]
                }
                frame "Spectrometer_Measure" {
                  w284 = "_"
                  n108 = Unbundle By Name(w253) -> ("Time Stamp"=w252:timestamp)
                  n109 = Unbundle By Name(w258) -> ("Wavlength"=w255:dbl[unit][])
                  n110 = property on="Measure_FileName" class="Str"() -> ("Value"=w283:string)  [unwired: 2 in, 2 out]
                  n111 = property on="Spectra Count" class="DigNum (strict)"() -> ("Value"=w288:u16)  [unwired: 2 in, 2 out]
                  n112 = Number To Decimal String(number=w288) -> (decimal integer string=w282:string)  [unwired: 1 in]
                  n113 = Format Date/Time String(time format string (%c)="%Y%m%d_%H%M%S", seconds (now)=w252) -> (date/time string=w285:string)  [unwired: 1 in]
                  n114 = Concatenate Strings(w285, w284, w283, w284, w282, ".spectra" ("string")) -> (w280:string)
                  n115 = property on="Measure_SavePath" class="Path"() -> ("Value"=w279:path)  [unwired: 2 in, 2 out]
                  n116 = Build Path(base path=w279, name or relative path=w280) -> (appended path=w278:path)
                  n117 = Unbundle By Name(w253) -> ("Data_Raw"=w273:T12)
                  n118 = Open/Create/Replace File(file path (use dialog)=w278, error in=w276, operation (0:open)=T11."open or create") -> (refnum out=w275:refnum<file>, error out=w274:errorcluster)  [unwired: 3 in, 1 out]
                  n119 = Index Array(array=w273, index=0) -> (element=w271:T13)
                  n120 = Unbundle By Name(w271) -> ("Image"=w259:dbl[][][])
                  n121 = Index Array(array=w259, index (dim 1)=0 ("disabled index (row)")) -> (element=w265:dbl[][])  [unwired: 2 in]
                  n122 = Transpose 2D Array(2D array=w265) -> (transposed array=w262:dbl[][])
                  n123 = To Unsigned Word Integer(number=w259) -> (unsigned 16bit integer=w270:u16[][][])
                  n124 = Matrix Size(0:w262) -> (2:w263:i32)  [unwired: 1 out]
                  n125 = Write to Binary File(file (use dialog)=w275, data=w270, error in=w274) -> (refnum out=w268:refnum<file>, error out=w269:errorcluster)  [unwired: 3 in, 1 out]
                  n126 = Reciprocal(x=w263) -> (1/x=w264:dbl)
                  n127 = Close File(refnum=w268, error in=w269) -> (error out=w267:errorcluster)  [unwired: 1 out]
                  n128 = Initialize Array(w264, w263) -> (w261:dbl[])
                  n129 = call-poly <vilib>:"A x B.vi"("Vector"=w261, "A"=w262) -> ("A x Vector"=w254:dbl[])  [unwired: 1 out]
                  n130 = Bundle("Wavlength"=w255, "A x Vector"=w254) -> (w257:T14)  [unwired: 1 in]
                  n131 = Build Array(w257) -> (w256:T15)
                  n132 = property on="Measure_Graph" class="XYGraph (strict)"("Value"=w256) -> ()  [unwired: 2 in, 2 out]
                }
                frame "Stop_Measurement" {
                  n133 = property on="Automatically \nadjust count" class="Bool (strict)"() -> ("Value"=w289:bool)  [unwired: 2 in, 2 out]
                  n134 = case shown="True" w289 {
                    frame False {
                    }
                    frame True {
                      n135 = Increment(x="Spectra Count") -> (x+1=w300:u16)
                      n136 = property on="Spectra Count" class="DigNum (strict)"("Value"=w300) -> ()  [unwired: 2 in, 2 out]
                    }
                  }
                  n137 = Get Queue Status(queue=w297) -> (queue out=w298:refnum<queue>, # elements in queue=w296:i32)  [unwired: 2 in, 6 out]
                  n138 = property on="Measure_MeasureSpectrum" class="Bool (strict)"("Value"=FALSE ("Measure Spectrum")) -> ()  [unwired: 2 in, 2 out]
                  n139 = for {
                    N: w296 -> [_]
                    shift-right: [w307] -> w293
                    shift-left: w298 -> [w308]
                    shift-right: [w304] -> w292
                    shift-left: w295 -> [w305]
                    shift-right: [w302] -> w291
                    shift-left: w294 -> [w303]
                    n140 = Dequeue Element(queue=w308) -> (queue out=w307:refnum<queue>, element=w306:T6)  [unwired: 2 in, 2 out]
                    n141 = Enqueue Element(queue=w305, element=w306, error in (no error)=w303) -> (queue out=w304:refnum<queue>, error out=w302:errorcluster)  [unwired: 1 in, 1 out]
                  }
                }
              }
            }
            n142 = Release Queue(queue=w226) -> ()  [unwired: 2 in, 3 out]
          }
          frame "Measure_SpectrumAdvanced" {
            w312 = T6 {"QueueAction"=enum."TimeOut", "Data"=[], "Data_Raw"=[], "Data_Dark"=[], "Data_Ref"=[], "Device Information"=[], "Numeric Control"=0.0, "Boolean"=FALSE, "Wavelength"=[], "Time"=[], "Time Stamp"=timestamp(0 s since 1904-01-01), "Numeric Control 2"=0.0, "TabControl"=enum."Measure"}  # DataQueue
            n143 = Obtain Queue(name (unnamed)="Temp", element data type=w312) -> (queue out=w311:refnum<queue>)  [unwired: 3 in, 2 out]
            n144 = while {
              shift-right: [w320] -> w315
              shift-left: w316 -> [w328]
              shift-right: [w321] -> w314
              shift-left: w317 -> [w329]
              shift-right: [w322] -> w310
              shift-left: w311 -> [w324]
              tunnel: w309 -> [w318]
              stop <- w319 stop-if-true
              n145 = Dequeue Element(queue=w328, error in (no error)=w329) -> (queue out=w326:refnum<queue>, element=w323:T6, error out=w325:errorcluster)  [unwired: 1 in, 1 out]
              n146 = Unbundle By Name(w323) -> ("QueueAction"=w327:T7)
              n147 = case shown="\"Spectrometer_Measure\"" w327 {
                tunnel: w326 -> [w330 w354 w380]
                tunnel: w325 -> [w333 w364 w379]
                tunnel: w324 -> [w335 w373 w382]
                tunnel: w323 -> [w331 w341 _]
                tunnel: [w334 w373 w378] -> w322
                tunnel: [w332 w355 w376] -> w321
                tunnel: [w330 w354 w377] -> w320
                tunnel: [_ _ TRUE] -> w319
                tunnel: w318 -> [_ w346 _]
                frame Default {
                  n148 = Enqueue Element(queue=w335, element=w331, error in (no error)=w333) -> (queue out=w334:refnum<queue>, error out=w332:errorcluster)  [unwired: 1 in, 1 out]
                }
                frame "Spectrometer_Measure" {
                  w370 = "_"
                  n149 = Unbundle By Name(w341) -> ("Time Stamp"=w340:timestamp)
                  n150 = property on="Nr After Spin" class="DigNum (strict)"() -> ("Value"=w339:u16)  [unwired: 2 in, 2 out]
                  n151 = Unbundle By Name(w346) -> ("Wavlength"=w343:dbl[unit][])
                  n152 = property on="Measure_FileName" class="Str"() -> ("Value"=w369:string)  [unwired: 2 in, 2 out]
                  n153 = Number To Decimal String(number=w339) -> (decimal integer string=w337:string)  [unwired: 1 in]
                  n154 = Format Date/Time String(time format string (%c)="%Y%m%d_%H%M%S", seconds (now)=w340) -> (date/time string=w371:string)  [unwired: 1 in]
                  n155 = Concatenate Strings(w371, w370, w369, w370, "a" ("string"), w337, ".spectra" ("string")) -> (w368:string)
                  n156 = property on="Measure_SavePath" class="Path"() -> ("Value"=w367:path)  [unwired: 2 in, 2 out]
                  n157 = Build Path(base path=w367, name or relative path=w368) -> (appended path=w366:path)
                  n158 = Unbundle By Name(w341) -> ("Data_Raw"=w361:T12)
                  n159 = Open/Create/Replace File(file path (use dialog)=w366, error in=w364, operation (0:open)=T11."open or create") -> (refnum out=w363:refnum<file>, error out=w362:errorcluster)  [unwired: 3 in, 1 out]
                  n160 = Index Array(array=w361, index=0) -> (element=w359:T13)
                  n161 = Unbundle By Name(w359) -> ("Image"=w347:dbl[][][])
                  n162 = Index Array(array=w347, index (dim 1)=0 ("disabled index (row)")) -> (element=w353:dbl[][])  [unwired: 2 in]
                  n163 = Transpose 2D Array(2D array=w353) -> (transposed array=w350:dbl[][])
                  n164 = To Unsigned Word Integer(number=w347) -> (unsigned 16bit integer=w358:u16[][][])
                  n165 = Matrix Size(0:w350) -> (2:w351:i32)  [unwired: 1 out]
                  n166 = Write to Binary File(file (use dialog)=w363, data=w358, error in=w362) -> (refnum out=w356:refnum<file>, error out=w357:errorcluster)  [unwired: 3 in, 1 out]
                  n167 = Reciprocal(x=w351) -> (1/x=w352:dbl)
                  n168 = Close File(refnum=w356, error in=w357) -> (error out=w355:errorcluster)  [unwired: 1 out]
                  n169 = Initialize Array(w352, w351) -> (w349:dbl[])
                  n170 = call-poly <vilib>:"A x B.vi"("Vector"=w349, "A"=w350) -> ("A x Vector"=w342:dbl[])  [unwired: 1 out]
                  n171 = Bundle("Wavlength"=w343, "A x Vector"=w342) -> (w345:T14)  [unwired: 1 in]
                  n172 = Build Array(w345) -> (w344:T15)
                  n173 = property on="Measure_Graph" class="XYGraph (strict)"("Value"=w344) -> ()  [unwired: 2 in, 2 out]
                }
                frame "Stop_Measurement" {
                  n174 = property on="Automatically \nadjust count" class="Bool (strict)"() -> ("Value"=w374:bool)  [unwired: 2 in, 2 out]
                  n175 = case shown="True" w374 {
                    frame False {
                    }
                    frame True {
                      n176 = property on="Nr After Spin" class="DigNum (strict)"() -> ("Value"=w386:u16)  [unwired: 2 in, 2 out]
                      n177 = Increment(x=w386) -> (x+1=w385:u16)
                      n178 = property on="Nr After Spin" class="DigNum (strict)"("Value"=w385) -> ()  [unwired: 2 in, 2 out]
                    }
                  }
                  n179 = Get Queue Status(queue=w382) -> (queue out=w383:refnum<queue>, # elements in queue=w381:i32)  [unwired: 2 in, 6 out]
                  n180 = property on="Measure_MeasureSpectrum" class="Bool (strict)"("Value"=FALSE ("Measure Spectrum")) -> ()  [unwired: 2 in, 2 out]
                  n181 = for {
                    N: w381 -> [_]
                    shift-right: [w392] -> w378
                    shift-left: w383 -> [w393]
                    shift-right: [w389] -> w377
                    shift-left: w380 -> [w390]
                    shift-right: [w387] -> w376
                    shift-left: w379 -> [w388]
                    n182 = Dequeue Element(queue=w393) -> (queue out=w392:refnum<queue>, element=w391:T6)  [unwired: 2 in, 2 out]
                    n183 = Enqueue Element(queue=w390, element=w391, error in (no error)=w388) -> (queue out=w389:refnum<queue>, error out=w387:errorcluster)  [unwired: 1 in, 1 out]
                  }
                }
              }
            }
            n184 = Release Queue(queue=w310) -> ()  [unwired: 2 in, 3 out]
          }
          frame "Save_InSitu" {
            w395 = "\r\n"
            w410 = 0 ("index (page)")
            n185 = Unbundle By Name(w434) -> ("Time Stamp"=w432:timestamp, "Device Information"=w423:string[], "Numeric Control"=w420:dbl, "Numeric Control 2"=w419:dbl)
            n186 = Unbundle By Name(w421) -> ("Dark"=w444:T12, "Ref"=w442:T12, "Wavlength"=w446:dbl[unit][])  [unwired: 1 out]
            n187 = node(w446) -> (w435:dbl[])
            n188 = property on="Frames" class="DigNum (strict)"() -> ("Value"=w406:i32)  [unwired: 2 in, 2 out]
            n189 = call "DeviceInfo2Str.vi"("Device Information"=w423) -> ("String"=w422:string)  [unwired: 10 in]
            n190 = Number To Decimal String(number=w406) -> (decimal integer string=w405:string)  [unwired: 1 in]
            n191 = property on="Seconds after Spin" class="DigNum (strict)"() -> ("Value"=w402:dbl[unit])  [unwired: 2 in, 2 out]
            n192 = property on="Seconds to Spin" class="DigNum (strict)"() -> ("Value"=w403:dbl[unit])  [unwired: 2 in, 2 out]
            n193 = Index Array(array=w442, index=0) -> (element=w440:T13)
            n194 = Index Array(array=w444, index=0) -> (element=w441:T13)
            n195 = property on="Measure_FileName" class="Str"() -> ("Value"=w416:string)  [unwired: 2 in, 2 out]
            n196 = property on="Program Spin Coater" class="Arr (strict)"() -> ("Value"=w404:T2)  [unwired: 2 in, 2 out]
            n197 = Unbundle By Name(w441) -> ("Image"=w439:dbl[][][])
            n198 = Unbundle By Name(w440) -> ("Image"=w438:dbl[][][])
            n199 = Format Date/Time String(time format string (%c)="%Y%m%d_%H%M%S", seconds (now)=w432) -> (date/time string=w431:string)  [unwired: 1 in]
            n200 = call "MeasurementSpin2String.vi"("Seconds after Spin Stop"=w402, "Seconds to Spin Start"=w403, "Program Spin Coater"=w404) -> ("concatenated string"=w401:string)
            n201 = Index Array(array=w438, index (dim 1)=w410) -> (element=w436:dbl[][])  [unwired: 2 in]
            n202 = Index Array(array=w439, index (dim 1)=w410) -> (element=w437:dbl[][])  [unwired: 2 in]
            n203 = property on="Duration after" class="DigNum (strict)"() -> ("Value"=w398:dbl[unit])  [unwired: 2 in, 2 out]
            n204 = Concatenate Strings(w431, "_" ("string"), w416) -> (w429:string)
            n205 = property on="periodic time" class="DigNum (strict)"() -> ("Value"=w399:dbl[unit])  [unwired: 2 in, 2 out]
            n206 = To Unsigned Word Integer(number=w437) -> (unsigned 16bit integer=w409:u16[][])
            n207 = property on="Spin at end" class="Bool (strict)"() -> ("Value"=w397:bool)  [unwired: 2 in, 2 out]
            n208 = To Unsigned Word Integer(number=w436) -> (unsigned 16bit integer=w408:u16[][])
            n209 = call "AfterSpinOptions.vi"("Spin at end"=w397, "Duration after"=w398, "periodic time"=w399) -> ("concatenated string"=w400:string)  [unwired: 8 in]
            n210 = Concatenate Strings(w422, w395, "Frames:\t" ("string"), w405, w395, w401, w395, w400, w395, "Comments:" ("string"), w395, "Measure_Comments") -> (w418:string)
            n211 = Bundle(w409, w408, w435, "Numeric Control"=w420, "Numeric Control 2"=w419) -> (w413:T16)  [unwired: 1 in]
            n212 = property on="Action" class="Str"("Value"="Saving" ("Action")) -> ()  [unwired: 2 in, 2 out]
            n213 = property on="Measure_SavePath" class="Path"() -> ("Value"=w415:path)  [unwired: 2 in, 2 out]
            n214 = Concatenate Strings(w429, "_add.spin" ("string")) -> (w427:string)
            n215 = Concatenate Strings(w429, "_comments.txt" ("string")) -> (w426:string)
            n216 = Build Path(base path=w415, name or relative path=w427) -> (appended path=w414:path)
            n217 = Build Path(base path=w415, name or relative path=w426) -> (appended path=w425:path)
            n218 = Write to Text File(file (use dialog)=w425, text=w418) -> (error out=w412:errorcluster)  [unwired: 2 in, 2 out]
            n219 = Write to Binary File(file (use dialog)=w414, data=w413) -> (error out=w411:errorcluster)  [unwired: 4 in, 2 out]
            n220 = flat-sequence {
              tunnel: w412 -> [_]
              tunnel: w411 -> [_]
              frame #0 {
                n221 = property on="Action" class="Str"("Value"="" ("Action")) -> ()  [unwired: 2 in, 2 out]
              }
            }
          }
          frame "Set_Dark" {
            # "Averaging"
            n222 = Unbundle By Name(w461) -> ("Wavlength"=w460:dbl[unit][])
            n223 = Unbundle By Name(w468) -> ("Data_Dark"=w458:T12)
            n224 = Index Array(array=w458, index=0) -> (element=w463:T13)
            n225 = Unbundle By Name(w463) -> ("Image"=w457:dbl[][][])
            n226 = Index Array(array=w457, index (dim 1)=0 ("disabled index (row)")) -> (element=w455:dbl[][])  [unwired: 2 in]
            n227 = Transpose 2D Array(2D array=w455) -> (transposed array=w452:dbl[][])
            n228 = Matrix Size(0:w452) -> (2:w453:i32)  [unwired: 1 out]
            n229 = Reciprocal(x=w453) -> (1/x=w454:dbl)
            n230 = Initialize Array(w454, w453) -> (w451:dbl[])
            n231 = call-poly <vilib>:"A x B.vi"("Vector"=w451, "A"=w452) -> ("A x Vector"=w450:dbl[])  [unwired: 1 out]
            n232 = Bundle("Wavlength"=w460, "A x Vector"=w450) -> (w462:T14)  [unwired: 1 in]
            n233 = Build Array(w462) -> (w459:T15)
            n234 = property on="Measure_Graph" class="XYGraph (strict)"("Value"=w459) -> ()  [unwired: 2 in, 2 out]
            n235 = Bundle By Name(cluster=w461, "Dark"=w458) -> (w465:T4)
          }
          frame "Set_Ref" {
            # "Averaging"
            n236 = Unbundle By Name(w470) -> ("Wavlength"=w469:dbl[unit][])
            n237 = Unbundle By Name(w487) -> ("Data_Ref"=w474:T12)
            n238 = Index Array(array=w474, index=0) -> (element=w482:T13)
            n239 = Unbundle By Name(w482) -> ("Image"=w481:dbl[][][])
            n240 = Index Array(array=w481, index (dim 1)=0 ("disabled index (row)")) -> (element=w479:dbl[][])  [unwired: 2 in]
            n241 = Transpose 2D Array(2D array=w479) -> (transposed array=w476:dbl[][])
            n242 = Matrix Size(0:w476) -> (2:w477:i32)  [unwired: 1 out]
            n243 = Reciprocal(x=w477) -> (1/x=w478:dbl)
            n244 = Initialize Array(w478, w477) -> (w475:dbl[])
            n245 = call-poly <vilib>:"A x B.vi"("Vector"=w475, "A"=w476) -> ("A x Vector"=w471:dbl[])  [unwired: 1 out]
            n246 = Bundle("Wavlength"=w469, "A x Vector"=w471) -> (w473:T14)  [unwired: 1 in]
            n247 = Build Array(w473) -> (w472:T15)
            n248 = Bundle By Name(cluster=w470, "Ref"=w474) -> (w484:T4)
            n249 = property on="Measure_Graph" class="XYGraph (strict)"("Value"=w472) -> ()  [unwired: 2 in, 2 out]
          }
          frame "Set_Wavelength" {
            n250 = Unbundle By Name(w490) -> ("Wavelength"=w493:dbl[unit][])
            n251 = Bundle By Name(cluster=w492, "Wavlength"=w493) -> (w491:T4)
          }
          frame "Spectrometer_Preview" {
            w498 = 0 ("index (page)")
            n252 = Unbundle By Name(w504) -> ("Data_Raw"=w502:T12)
            n253 = Unbundle By Name(w503) -> ("Wavlength"=w497:dbl[unit][])
            n254 = Index Array(array=w502, index=0) -> (element=w500:T13)
            n255 = Unbundle By Name(w500) -> ("Image"=w499:dbl[][][])
            n256 = Index Array(array=w499, index (dim 0)=w498, index (dim 1)=w498) -> (element=w496:dbl[])  [unwired: 1 in]
            n257 = Bundle("Wavlength"=w497, "Image"=w496) -> (w495:cluster{"Wavlength":dbl[unit][], "Image":dbl[]})  [unwired: 1 in]
            n258 = Build Array(w495) -> (→"Measure_Graph":T3)
          }
        }
      }
      frame Error {
        w512 = T17 4 items=["no dialog", "OK message", "continue or stop message", "OK message + warnings", "continue/stop + warnings"] ("type of dialog (OK msg:1)")
        n259 = call <vilib>:"General Error Handler.vi"("type of dialog (OK msg:1)"=w512, "error in (no error)"=w509) -> ("error out"=w511:errorcluster)  [unwired: 9 in, 4 out]
        n260 = call <vilib>:"Clear Errors.vi"("error in (no error)"=w511) -> ("error out"=w508:errorcluster)  [unwired: 5 in, 1 out]
      }
    }
  }
  n261 = while {
    shift-right: [w515] -> _
    shift-left: w12 -> [w513]
    shift-right: [w518] -> _
    shift-left: w7 -> [w519]
    shift-right: [w516] -> _
    shift-left: w8 -> [w517]
    stop <- w514 stop-if-true
    # "Producer"
    n262 = event shown="[1] \"Stop Button\": Value Change" {
      selector: _ -> [_ _ _ _ _ _ _ _ _ _ _ _ _ _ _ _ _ _ _ _ _]
      dyn-events: _ -> [_ _ _ _ _ _ _ _ _ _ _ _ _ _ _ _ _ _ _ _ _]
      timeout: -1 -> [_ _ _ _ _ _ _ _ _ _ _ _ _ _ _ _ _ _ _ _ _]
      tunnel: w519 -> [w522 w537 w541 w553 w566 w581 w593 w604 w607 w614 w633 w640 w649 w657 w672 w682 w691 w699 w704 w712 w723]
      tunnel: [w522 w534 w541 w553 w566 w581 w593 w604 w607 w614 w633 w640 w649 w656 w672 w682 w691 w699 w704 w710 w723] -> w518
      tunnel: w517 -> [w521 w536 w543 w551 w563 w580 w591 w599 w606 w611 w631 w639 w647 w663 w669 w681 w690 w698 w703 w716 w724]
      tunnel: [w521 w530 w540 w547 w562 w578 w589 w598 w606 w609 w630 w637 w646 w655 w670 w678 w687 w698 w703 w716 w724] -> w516
      tunnel: w513 -> [w523 w538 w544 w552 w565 w582 w592 w601 w608 w612 w634 w641 w650 w665 w673 w683 w692 w700 w705 w717 w722]
      tunnel: [w523 w535 w542 w548 w564 w579 w590 w600 w608 w613 w632 w638 w648 w664 w671 w679 w688 w700 w702 w715 w722] -> w515
      tunnel: [_ TRUE _ _ _ _ _ _ _ _ _ _ _ _ _ _ _ _ _ _ _] -> w514
      event Timeout {
        n263 = event-data() -> ()  [unwired: 1 in, 3 out]
      }
      event "Stop Button": Value Change {
        w526 = T6 {"QueueAction"=enum."TimeOut", "Data"=[], "Data_Raw"=[], "Data_Dark"=[], "Data_Ref"=[], "Device Information"=[], "Numeric Control"=0.0, "Boolean"=FALSE, "Wavelength"=[], "Time"=[], "Time Stamp"=timestamp(0 s since 1904-01-01), "Numeric Control 2"=0.0, "TabControl"=enum."Measure"}  # DataQueue
        w529 = T9 {"QueueAction"=enum."TimeOut", "Numeric 1"=0.0, "Numeric 2"=0.0, "Boolean 1"=FALSE, "Boolean 2"=FALSE, "Spin Program"=[], "Spin Prg v07"=[], "Time Stamp"=timestamp(0 s since 1904-01-01), "TabControl"=enum."Measure"}  # Device Queue
        n264 = event-data() -> ()  [unwired: 1 in, 6 out]
        n265 = Bundle By Name(cluster=w529, "QueueAction"=DeviceQueue_Action."Close_Program") -> (w527:T9)
        n266 = Enqueue Element(queue=w538, element=w527, error in (no error)=w536) -> (queue out=w535:refnum<queue>, error out=w531:errorcluster)  [unwired: 1 in, 1 out]
        n267 = Bundle By Name(cluster=w526, "QueueAction"=DataQueue_Action."Close_Program") -> (w524:T6)
        n268 = Enqueue Element(queue=w537, element=w524, error in (no error)=w536) -> (queue out=w534:refnum<queue>, error out=w532:errorcluster)  [unwired: 1 in, 1 out]
        n269 = Merge Errors(w532, w531) -> (w530:errorcluster)
      }
      event "Abort Button": Value Change {
        w546 = T9 {"QueueAction"=enum."TimeOut", "Numeric 1"=0.0, "Numeric 2"=0.0, "Boolean 1"=FALSE, "Boolean 2"=FALSE, "Spin Program"=[], "Spin Prg v07"=[], "Time Stamp"=timestamp(0 s since 1904-01-01), "TabControl"=enum."Measure"}  # Device Queue
        # "At the moment just spin coater in non in-situ measurements can be stopped"
        n270 = event-data() -> ()  [unwired: 1 in, 6 out]
        n271 = Bundle By Name(cluster=w546, "QueueAction"=DeviceQueue_Action."Abort") -> (w545:T9)
        n272 = Enqueue Element(queue=w544, element=w545, error in (no error)=w543) -> (queue out=w542:refnum<queue>, error out=w540:errorcluster)  [unwired: 1 in, 1 out]
      }
      event "Init_Spectrometer": Value Change {
        n273 = event-data() -> ()  [unwired: 1 in, 6 out]
        n274 = case shown="True" "Init_Spectrometer" {
          tunnel: [w554 w557] -> w549
          frame True {
            n275 = Bundle By Name(cluster=T9 {"QueueAction"=enum."TimeOut", "Numeric 1"=0.0, "Numeric 2"=0.0, "Boolean 1"=FALSE, "Boolean 2"=FALSE, "Spin Program"=[], "Spin Prg v07"=[], "Time Stamp"=timestamp(0 s since 1904-01-01), "TabControl"=enum."Measure"} ("element"), "QueueAction"=DeviceQueue_Action."Spectrometer_Init") -> (w554:T9)
          }
          frame False {
            n276 = Bundle By Name(cluster=T9 {"QueueAction"=enum."TimeOut", "Numeric 1"=0.0, "Numeric 2"=0.0, "Boolean 1"=FALSE, "Boolean 2"=FALSE, "Spin Program"=[], "Spin Prg v07"=[], "Time Stamp"=timestamp(0 s since 1904-01-01), "TabControl"=enum."Measure"} ("element"), "QueueAction"=DeviceQueue_Action."Spectrometer_Close") -> (w557:T9)
          }
        }
        n277 = Enqueue Element(queue=w552, element=w549, error in (no error)=w551) -> (queue out=w548:refnum<queue>, error out=w547:errorcluster)  [unwired: 1 in, 1 out]
      }
      event "Init_Arduino": Value Change {
        n278 = event-data() -> ("NewVal"=w561:bool)  [unwired: 1 in, 5 out]
        n279 = case shown="True" w561 {
          tunnel: [w567 w570] -> w560
          frame False {
            w569 = T9 {"QueueAction"=enum."TimeOut", "Numeric 1"=0.0, "Numeric 2"=0.0, "Boolean 1"=FALSE, "Boolean 2"=FALSE, "Spin Program"=[], "Spin Prg v07"=[], "Time Stamp"=timestamp(0 s since 1904-01-01), "TabControl"=enum."Measure"}  # Device Queue
            n280 = Bundle By Name(cluster=w569, "QueueAction"=DeviceQueue_Action."Arduino_Close") -> (w567:T9)
          }
          frame True {
            w572 = T9 {"QueueAction"=enum."TimeOut", "Numeric 1"=0.0, "Numeric 2"=0.0, "Boolean 1"=FALSE, "Boolean 2"=FALSE, "Spin Program"=[], "Spin Prg v07"=[], "Time Stamp"=timestamp(0 s since 1904-01-01), "TabControl"=enum."Measure"}  # Device Queue
            n281 = Bundle By Name(cluster=w572, "QueueAction"=DeviceQueue_Action."Arduino_Init") -> (w570:T9)
          }
        }
        n282 = Enqueue Element(queue=w565, element=w560, error in (no error)=w563) -> (queue out=w564:refnum<queue>, error out=w562:errorcluster)  [unwired: 1 in, 1 out]
      }
      event "Program Spin Coater": Value Change {
        w584 = T9 {"QueueAction"=enum."TimeOut", "Numeric 1"=0.0, "Numeric 2"=0.0, "Boolean 1"=FALSE, "Boolean 2"=FALSE, "Spin Program"=[], "Spin Prg v07"=[], "Time Stamp"=timestamp(0 s since 1904-01-01), "TabControl"=enum."Measure"}  # Device Queue
        n283 = event-data() -> ("NewVal"=w573:T2)  [unwired: 1 in, 5 out]
        n284 = property on="Seconds to Spin" class="DigNum (strict)"() -> ("Value"=w575:dbl[unit])  [unwired: 2 in, 2 out]
        n285 = node(w575) -> (w574:dbl)
        n286 = Bundle By Name(cluster=w584, "QueueAction"=DeviceQueue_Action."Arduino_LoadProgram", "Spin Prg v07"=w573, "Numeric 1"=w574) -> (w583:T9)
        n287 = Enqueue Element(queue=w582, element=w583, error in (no error)=w580) -> (queue out=w579:refnum<queue>, error out=w578:errorcluster)  [unwired: 1 in, 1 out]
        n288 = property on="Measure_IntegrationTime" class="DigNum (strict)"() -> ("Value"=w576:dbl[unit])  [unwired: 2 in, 2 out]
        n289 = property on="Measure_IntegrationTime" class="DigNum (strict)"("Val(Sgnl)"=w576) -> ()  [unwired: 2 in, 2 out]
      }
      event "Measure_IntegrationTime": Value Change {
        w595 = T9 {"QueueAction"=enum."TimeOut", "Numeric 1"=0.0, "Numeric 2"=0.0, "Boolean 1"=FALSE, "Boolean 2"=FALSE, "Spin Program"=[], "Spin Prg v07"=[], "Time Stamp"=timestamp(0 s since 1904-01-01), "TabControl"=enum."Measure"}  # Device Queue
        n290 = event-data() -> ("NewVal"=w587:dbl[unit])  [unwired: 1 in, 5 out]
        n291 = node(w587) -> (w586:dbl)
        n292 = property on="Calculate Frames" class="Bool (strict)"() -> ("Value"=w585:bool)  [unwired: 2 in, 2 out]
        n293 = Bundle By Name(cluster=w595, "QueueAction"=DeviceQueue_Action."Spectrometer_SetIntegrationTime", "Numeric 1"=w586, "Boolean 1"=w585) -> (w594:T9)
        n294 = Enqueue Element(queue=w592, element=w594, error in (no error)=w591) -> (queue out=w590:refnum<queue>, error out=w589:errorcluster)  [unwired: 1 in, 1 out]
      }
      event "Frames": Value Change {
        w603 = T9 {"QueueAction"=enum."TimeOut", "Numeric 1"=0.0, "Numeric 2"=0.0, "Boolean 1"=FALSE, "Boolean 2"=FALSE, "Spin Program"=[], "Spin Prg v07"=[], "Time Stamp"=timestamp(0 s since 1904-01-01), "TabControl"=enum."Measure"}  # Device Queue
        n295 = event-data() -> ()  [unwired: 1 in, 6 out]
        n296 = Bundle By Name(cluster=w603, "QueueAction"=DeviceQueue_Action."Spectrometer_SetFrames", "Numeric 1"="Frames") -> (w602:T9)
        n297 = Enqueue Element(queue=w601, element=w602, error in (no error)=w599) -> (queue out=w600:refnum<queue>, error out=w598:errorcluster)  [unwired: 1 in, 1 out]
      }
      event "Seconds to Spin", "Seconds after Spin": Value Change {
        n298 = event-data() -> ()  [unwired: 1 in, 6 out]
        n299 = property on="Program Spin Coater" class="Arr (strict)"() -> ("Value"=w605:T2)  [unwired: 2 in, 2 out]
        n300 = property on="Program Spin Coater" class="Arr (strict)"("Val(Sgnl)"=w605) -> ()  [unwired: 2 in, 2 out]
      }
      event "Calculate Frames": Value Change {
        n301 = event-data() -> ("NewVal"=w615:bool)  [unwired: 1 in, 5 out]
        n302 = case shown="False" w615 {
          tunnel: [0 2] -> w610
          tunnel: w612 -> [w617 w626]
          tunnel: [w617 w624] -> w613
          tunnel: w611 -> [w616 w623]
          tunnel: [w616 w619] -> w609
          frame False {
          }
          frame True {
            w625 = T9 {"QueueAction"=enum."TimeOut", "Numeric 1"=0.0, "Numeric 2"=0.0, "Boolean 1"=FALSE, "Boolean 2"=FALSE, "Spin Program"=[], "Spin Prg v07"=[], "Time Stamp"=timestamp(0 s since 1904-01-01), "TabControl"=enum."Measure"}  # Device Queue
            n303 = property on="Measure_IntegrationTime" class="DigNum (strict)"() -> ("Value"=w621:dbl[unit])  [unwired: 2 in, 2 out]
            n304 = node(w621) -> (w620:dbl)
            n305 = Bundle By Name(cluster=w625, "QueueAction"=DeviceQueue_Action."Spectrometer_SetIntegrationTime", "Numeric 1"=w620) -> (w627:T9)
            n306 = Enqueue Element(queue=w626, element=w627, error in (no error)=w623) -> (queue out=w624:refnum<queue>, error out=w619:errorcluster)  [unwired: 1 in, 1 out]
          }
        }
        n307 = property on="Frames" class="DigNum (strict)"("DisabledEnum"=w610) -> ()  [unwired: 2 in, 2 out]
      }
      event "Record RefSpec": Value Change {
        w636 = T9 {"QueueAction"=enum."TimeOut", "Numeric 1"=0.0, "Numeric 2"=0.0, "Boolean 1"=FALSE, "Boolean 2"=FALSE, "Spin Program"=[], "Spin Prg v07"=[], "Time Stamp"=timestamp(0 s since 1904-01-01), "TabControl"=enum."Measure"}  # Device Queue
        n308 = event-data() -> ()  [unwired: 1 in, 6 out]
        n309 = Bundle By Name(cluster=w636, "QueueAction"=DeviceQueue_Action."Spectrometer_SetReference") -> (w635:T9)
        n310 = Enqueue Element(queue=w634, element=w635, error in (no error)=w631) -> (queue out=w632:refnum<queue>, error out=w630:errorcluster)  [unwired: 1 in, 1 out]
      }
      event "Measure_Preview": Value Change {
        w644 = T9 {"QueueAction"=enum."TimeOut", "Numeric 1"=0.0, "Numeric 2"=0.0, "Boolean 1"=FALSE, "Boolean 2"=FALSE, "Spin Program"=[], "Spin Prg v07"=[], "Time Stamp"=timestamp(0 s since 1904-01-01), "TabControl"=enum."Measure"}  # Device Queue
        n311 = event-data() -> ()  [unwired: 1 in, 6 out]
        n312 = Bundle By Name(cluster=w644, "QueueAction"=DeviceQueue_Action."Spectrometer_Preview") -> (w643:T9)
        n313 = Enqueue Element(queue=w641, element=w643, error in (no error)=w639) -> (queue out=w638:refnum<queue>, error out=w637:errorcluster)  [unwired: 1 in, 1 out]
      }
      event "Record_Darkspec": Value Change {
        w652 = T9 {"QueueAction"=enum."TimeOut", "Numeric 1"=0.0, "Numeric 2"=0.0, "Boolean 1"=FALSE, "Boolean 2"=FALSE, "Spin Program"=[], "Spin Prg v07"=[], "Time Stamp"=timestamp(0 s since 1904-01-01), "TabControl"=enum."Measure"}  # Device Queue
        n314 = event-data() -> ()  [unwired: 1 in, 6 out]
        n315 = Bundle By Name(cluster=w652, "QueueAction"=DeviceQueue_Action."Spectrometer_SetDarkspec") -> (w651:T9)
        n316 = Enqueue Element(queue=w650, element=w651, error in (no error)=w647) -> (queue out=w648:refnum<queue>, error out=w646:errorcluster)  [unwired: 1 in, 1 out]
      }
      event "StartMeasurement_Button": Value Change {
        w659 = T6 {"QueueAction"=enum."TimeOut", "Data"=[], "Data_Raw"=[], "Data_Dark"=[], "Data_Ref"=[], "Device Information"=[], "Numeric Control"=0.0, "Boolean"=FALSE, "Wavelength"=[], "Time"=[], "Time Stamp"=timestamp(0 s since 1904-01-01), "Numeric Control 2"=0.0, "TabControl"=enum."Measure"}  # DataQueue
        w667 = T9 {"QueueAction"=enum."TimeOut", "Numeric 1"=0.0, "Numeric 2"=0.0, "Boolean 1"=FALSE, "Boolean 2"=FALSE, "Spin Program"=[], "Spin Prg v07"=[], "Time Stamp"=timestamp(0 s since 1904-01-01), "TabControl"=enum."Measure"}  # Device Queue
        n317 = event-data() -> ()  [unwired: 1 in, 6 out]
        n318 = property on="Measure_Preview" class="Bool (strict)"("Value"=FALSE ("Preview")) -> ()  [unwired: 2 in, 2 out]
        n319 = Get Date/Time In Seconds() -> (seconds since 1Jan1904=w653:timestamp)
        n320 = Bundle By Name(cluster=w667, "QueueAction"=DeviceQueue_Action."Measure_InSituAdvanced", "Time Stamp"=w653) -> (w666:T9)
        n321 = Enqueue Element(queue=w665, element=w666, error in (no error)=w663) -> (queue out=w664:refnum<queue>, error out=w654:errorcluster)  [unwired: 1 in, 1 out]
        n322 = Bundle By Name(cluster=w659, "QueueAction"=DataQueue_Action."Measure_InSituSpinCoating", "Time Stamp"=w653) -> (w660:T6)
        n323 = Enqueue Element(queue=w657, element=w660, error in (no error)=w654) -> (queue out=w656:refnum<queue>, error out=w655:errorcluster)  [unwired: 1 in, 1 out]
      }
      event "StartSpin_Button": Value Change {
        w675 = T9 {"QueueAction"=enum."TimeOut", "Numeric 1"=0.0, "Numeric 2"=0.0, "Boolean 1"=FALSE, "Boolean 2"=FALSE, "Spin Program"=[], "Spin Prg v07"=[], "Time Stamp"=timestamp(0 s since 1904-01-01), "TabControl"=enum."Measure"}  # Device Queue
        n324 = event-data() -> ()  [unwired: 1 in, 6 out]
        n325 = Bundle By Name(cluster=w675, "QueueAction"=DeviceQueue_Action."Arduino_StartProgram") -> (w674:T9)
        n326 = Enqueue Element(queue=w673, element=w674, error in (no error)=w669) -> (queue out=w671:refnum<queue>, error out=w670:errorcluster)  [unwired: 1 in, 1 out]
      }
      event "Milliseconds": Value Change {
        w684 = T9 {"QueueAction"=enum."TimeOut", "Numeric 1"=0.0, "Numeric 2"=0.0, "Boolean 1"=FALSE, "Boolean 2"=FALSE, "Spin Program"=[], "Spin Prg v07"=[], "Time Stamp"=timestamp(0 s since 1904-01-01), "TabControl"=enum."Measure"}  # Device Queue
        n327 = event-data() -> ()  [unwired: 1 in, 6 out]
        n328 = Bundle By Name(cluster=w684, "QueueAction"=DeviceQueue_Action."Arduino_SetMillis", "Numeric 1"="Milliseconds") -> (w680:T9)
        n329 = Enqueue Element(queue=w683, element=w680, error in (no error)=w681) -> (queue out=w679:refnum<queue>, error out=w678:errorcluster)  [unwired: 1 in, 1 out]
      }
      event "Speed": Value Change {
        w693 = T9 {"QueueAction"=enum."TimeOut", "Numeric 1"=0.0, "Numeric 2"=0.0, "Boolean 1"=FALSE, "Boolean 2"=FALSE, "Spin Program"=[], "Spin Prg v07"=[], "Time Stamp"=timestamp(0 s since 1904-01-01), "TabControl"=enum."Measure"}  # Device Queue
        n330 = event-data() -> ()  [unwired: 1 in, 6 out]
        n331 = Bundle By Name(cluster=w693, "QueueAction"=DeviceQueue_Action."Arduino_SetSpeed", "Numeric 1"="Speed") -> (w689:T9)
        n332 = Enqueue Element(queue=w692, element=w689, error in (no error)=w690) -> (queue out=w688:refnum<queue>, error out=w687:errorcluster)  [unwired: 1 in, 1 out]
      }
      event "Debug": Value Change {
        n333 = event-data() -> ()  [unwired: 1 in, 6 out]
        n334 = Select(t=u8 0, s="Debug", f=u8 2) -> (s? t:f=w694:u8)
        n335 = property on="Milliseconds" class="DigNum (strict)"("DisabledEnum"=w694) -> ()  [unwired: 2 in, 2 out]
        n336 = property on="Speed" class="DigNum (strict)"("DisabledEnum"=w694) -> ()  [unwired: 2 in, 2 out]
      }
      event "Measure_FramesSpectrometer": Value Change {
        w707 = T9 {"QueueAction"=enum."TimeOut", "Numeric 1"=0.0, "Numeric 2"=0.0, "Boolean 1"=FALSE, "Boolean 2"=FALSE, "Spin Program"=[], "Spin Prg v07"=[], "Time Stamp"=timestamp(0 s since 1904-01-01), "TabControl"=enum."Measure"}  # Device Queue
        n337 = event-data() -> ("NewVal"=w701:dbl)  [unwired: 1 in, 5 out]
        n338 = Bundle By Name(cluster=w707, "QueueAction"=DeviceQueue_Action."Spectrometer_SetFrames", "Numeric 1"=w701) -> (w708:T9)
        n339 = Enqueue Element(queue=w705, element=w708) -> (queue out=w702:refnum<queue>)  [unwired: 2 in, 2 out]
      }
      event "Measure_MeasureSpectrum": Value Change {
        w714 = T6 {"QueueAction"=enum."TimeOut", "Data"=[], "Data_Raw"=[], "Data_Dark"=[], "Data_Ref"=[], "Device Information"=[], "Numeric Control"=0.0, "Boolean"=FALSE, "Wavelength"=[], "Time"=[], "Time Stamp"=timestamp(0 s since 1904-01-01), "Numeric Control 2"=0.0, "TabControl"=enum."Measure"}  # DataQueue
        w719 = T9 {"QueueAction"=enum."TimeOut", "Numeric 1"=0.0, "Numeric 2"=0.0, "Boolean 1"=FALSE, "Boolean 2"=FALSE, "Spin Program"=[], "Spin Prg v07"=[], "Time Stamp"=timestamp(0 s since 1904-01-01), "TabControl"=enum."Measure"}  # Device Queue
        n340 = event-data() -> ()  [unwired: 1 in, 6 out]
        n341 = Get Date/Time In Seconds() -> (seconds since 1Jan1904=w709:timestamp)
        n342 = Bundle By Name(cluster=w719, "QueueAction"=DeviceQueue_Action."Measure_Spectrum", "Time Stamp"=w709) -> (w720:T9)
        n343 = Enqueue Element(queue=w717, element=w720) -> (queue out=w715:refnum<queue>)  [unwired: 2 in, 2 out]
        n344 = Bundle By Name(cluster=w714, "QueueAction"=DataQueue_Action."Measure_Spectrum") -> (w711:T6)
        n345 = Enqueue Element(queue=w712, element=w711) -> (queue out=w710:refnum<queue>)  [unwired: 2 in, 2 out]
      }
      event "Automatically \nadjust count": Value Change {
        n346 = event-data() -> ("NewVal"=w727:bool)  [unwired: 1 in, 5 out]
        n347 = Select(t=u8 2, s=w727, f=u8 0) -> (s? t:f=w721:u8)
        n348 = property on="Spectra Count" class="DigNum (strict)"("DisabledEnum"=w721) -> ()  [unwired: 2 in, 2 out]
      }
    }
  }
  n349 = while {
    shift-right: [w732] -> _
    shift-left: w8 -> [w736]
    shift-right: [w733] -> w10
    shift-left: w12 -> [w735]
    shift-right: [w730] -> w9
    shift-left: w7 -> [w731]
    shift-right: [w728] -> _
    shift-left: w11 -> [w729]
    stop <- w734 stop-if-true
    # "Consumer Devices"
    n350 = case shown="No Error" w736 {
      selector: w736 -> [w749 w1346]
      tunnel: w735 -> [w750 w1347]
      tunnel: [w746 _] -> w734
      tunnel: [w745 w1347] -> w733
      tunnel: [w743 w1343] -> w732
      tunnel: w731 -> [w741 w1341]
      tunnel: [w742 w1341] -> w730
      tunnel: w729 -> [w740 w1342]
      tunnel: [w739 w1342] -> w728
      frame No Error {
        n351 = Dequeue Element(queue=w750, timeout in ms (-1)=100, error in (no error)=w749) -> (queue out=w748:refnum<queue>, element=w738:T9, error out=w744:errorcluster)  [unwired: 1 out]
        n352 = Unbundle By Name(w738) -> ("QueueAction"=w747:T10)
        n353 = case shown="\"Spectrometer_MeasureAdvanced\"" w747 {
          tunnel: w748 -> [w755 w760 w784 w802 w811 w861 w877 w902 w911 w930 w937 w956 w957 w985 w1002 w1017 w1027 w1039 w1051 w1072 w1094 w1099 w1106 w1118 w1124 w1134 w1180 w1270 w1338]
          tunnel: [_ _ w786 _ _ _ _ _ _ _ _ _ _ _ _ _ _ _ _ _ _ _ _ _ _ _ _ _ _] -> w746
          tunnel: [w755 w760 w769 w788 w810 w861 w877 w902 w912 w930 w937 w956 w957 w985 w1002 w1017 w1027 w1039 w1050 w1072 w1094 w1099 w1106 w1118 w1124 w1134 w1142 w1196 w1329] -> w745
          tunnel: w744 -> [w754 w759 w768 w801 w822 w862 w876 w901 w907 w933 w941 w953 w967 w983 w992 w1008 w1024 w1035 w1046 w1075 w1088 w1096 w1104 w1113 w1121 w1127 w1136 w1231 w1337]
          tunnel: [w754 w759 w767 w789 w809 w856 w875 w900 w905 w931 w938 w943 w961 w982 w989 w1004 w1022 w1029 w1049 w1074 w1085 w1095 w1102 w1112 w1120 w1126 w1143 w1197 w1328] -> w743
          tunnel: [w752 w757 w766 w806 w807 w858 w868 w882 w916 w929 w936 w947 w969 w986 w996 w1011 w1018 w1031 w1053 w1073 w1093 w1101 w1110 w1116 w1125 w1129 w1151 w1243 w1336] -> w742
          tunnel: w741 -> [w752 w757 w766 w806 w808 w858 w867 w891 w917 w929 w936 w948 w969 w986 w999 w1014 w1018 w1033 w1053 w1073 w1093 w1101 w1110 w1116 w1125 w1130 w1151 w1243 w1336]
          tunnel: w740 -> [w753 w758 w765 w805 w819 w860 w874 w899 w910 w928 w940 w949 w960 w979 w995 w1010 w1021 w1028 w1048 w1068 w1087 w1100 w1109 w1115 w1123 w1128 w1183 w1273 w1335]
          tunnel: [w753 w758 w765 w805 w813 w859 w874 w899 w909 w926 w935 w949 w958 w980 w994 w1009 w1019 w1028 w1052 w1066 w1084 w1100 w1109 w1115 w1123 w1128 w1183 w1273 w1335] -> w739
          tunnel: w738 -> [_ w764 _ _ _ _ w866 w893 _ _ _ w955 w964 w987 _ _ w1025 _ _ _ w1092 _ w1108 w1117 _ _ _ w1213 w1327]
          frame "TimeOut", Default {
            n354 = property on="Action" class="Str"("Value"="TimeOut" ("Action")) -> ()  [unwired: 2 in, 2 out]
          }
          frame "Wait" {
            n355 = Unbundle By Name(w764) -> ("Numeric 1"=w763:dbl)
            n356 = Multiply(x=w763, y=1000.0) -> (x*y=w761:dbl)
            n357 = Wait (ms)(milliseconds to wait=w761) -> ()  [unwired: 1 out]
            n358 = property on="Action" class="Str"("Value"="Wait" ("Action")) -> ()  [unwired: 2 in, 2 out]
          }
          frame "Close_Program" {
            w785 = T9 {"QueueAction"=enum."TimeOut", "Numeric 1"=0.0, "Numeric 2"=0.0, "Boolean 1"=FALSE, "Boolean 2"=FALSE, "Spin Program"=[], "Spin Prg v07"=[], "Time Stamp"=timestamp(0 s since 1904-01-01), "TabControl"=enum."Measure"}  # Device Queue
            n359 = Bundle By Name(cluster=w785, "QueueAction"=DeviceQueue_Action."Spectrometer_Close") -> (w780:T9)
            n360 = Bundle By Name(cluster=w780, "QueueAction"=DeviceQueue_Action."Laser_Close") -> (w778:T9)
            n361 = Bundle By Name(cluster=w778, "QueueAction"=DeviceQueue_Action."Arduino_Close") -> (w772:T9)
            n362 = Enqueue Element(queue=w784, element=w780, error in (no error)=w768) -> (queue out=w782:refnum<queue>, error out=w777:errorcluster)  [unwired: 1 in, 1 out]
            n363 = Bundle By Name(cluster=w772, "QueueAction"=DeviceQueue_Action."Close_Program") -> (w770:T9)
            n364 = Enqueue Element(queue=w782, element=w778, error in (no error)=w777) -> (queue out=w776:refnum<queue>, error out=w775:errorcluster)  [unwired: 1 in, 1 out]
            n365 = Enqueue Element(queue=w776, element=w772, error in (no error)=w775) -> (queue out=w774:refnum<queue>, error out=w773:errorcluster)  [unwired: 1 in, 1 out]
            n366 = Enqueue Element(queue=w774, element=w770, error in (no error)=w773) -> (queue out=w769:refnum<queue>, error out=w767:errorcluster)  [unwired: 1 in, 1 out]
            n367 = First Call?() -> (First Call?: T/F=w787:bool)
            n368 = Not(x=w787) -> (.not. x?=w786:bool)
          }
          frame "Abort" {
            w804 = T9 {"QueueAction"=enum."TimeOut", "Numeric 1"=0.0, "Numeric 2"=0.0, "Boolean 1"=FALSE, "Boolean 2"=FALSE, "Spin Program"=[], "Spin Prg v07"=[], "Time Stamp"=timestamp(0 s since 1904-01-01), "TabControl"=enum."Measure"}  # Device Queue
            n369 = Flush Queue(queue=w802, error in (no error)=w801) -> (queue out=w800:refnum<queue>, error out=w799:errorcluster)  [unwired: 1 out]
            n370 = Bundle By Name(cluster=w804, "QueueAction"=DeviceQueue_Action."Spectrometer_StopMeasurement") -> (w796:T9)
            n371 = Bundle By Name(cluster=w796, "QueueAction"=DeviceQueue_Action."Arduino_StopSpin") -> (w792:T9)
            n372 = Enqueue Element(queue=w800, element=w796, error in (no error)=w799) -> (queue out=w798:refnum<queue>, error out=w797:errorcluster)  [unwired: 1 in, 1 out]
            n373 = Bundle By Name(cluster=w792, "QueueAction"=DeviceQueue_Action."Measure_Stop") -> (w791:T9)
            n374 = Enqueue Element(queue=w798, element=w792, error in (no error)=w797) -> (queue out=w794:refnum<queue>, error out=w793:errorcluster)  [unwired: 1 in, 1 out]
            n375 = Enqueue Element(queue=w794, element=w791, error in (no error)=w793) -> (queue out=w788:refnum<queue>, error out=w789:errorcluster)  [unwired: 1 in, 1 out]
          }
          frame "Spectrometer_Init" {
            n376 = call-dynamic "Init.vi"("error in (no error)"=w822, "Variant"=0, "Avantes in"=refnum<class "Avantes.lvclass"> refnum ("Avantes.lvclass")) -> ("error out"=w821:errorcluster, "Avantes out"=w820:refnum<class "Avantes.lvclass">)  [unwired: 7 in]
            n377 = call-dynamic "IsInit.vi"("error in (no error)"=w821, "Avantes in"=w820) -> ("error out"=w817:errorcluster, "Is Init?"=w816:bool, "Avantes out"=w818:refnum<class "Avantes.lvclass">)  [unwired: 7 in]
            n378 = property on="Spectromter" class="Bool (strict)"("Value"=w816) -> ()  [unwired: 2 in, 2 out]
            n379 = property on="Init_Spectrometer" class="Bool (strict)"("Value"=w816) -> ()  [unwired: 2 in, 2 out]
            n380 = call-dynamic "Set_ExposurePerFrame.vi"("error in (no error)"=w817, "Exposure per Frame"=1, "Avantes in"=w818) -> ("error out"=w812:errorcluster, "Avantes out"=w815:refnum<class "Avantes.lvclass">)  [unwired: 7 in]
            n381 = case shown="True" w816 {
              tunnel: w815 -> [_ w838]
              tunnel: w812 -> [w827 w836]
              tunnel: [refnum<class "Abstract_CCD.lvclass"> refnum ("Abstract_CCD.lvclass") w837] -> w814
              tunnel: w811 -> [w828 w853]
              tunnel: [w828 w842] -> w810
              tunnel: [w827 w841] -> w809
              tunnel: w808 -> [w826 w833]
              tunnel: [w826 w831] -> w807
              frame False {
              }
              frame True {
                w839 = T6 {"QueueAction"=enum."TimeOut", "Data"=[], "Data_Raw"=[], "Data_Dark"=[], "Data_Ref"=[], "Device Information"=[], "Numeric Control"=0.0, "Boolean"=FALSE, "Wavelength"=[], "Time"=[], "Time Stamp"=timestamp(0 s since 1904-01-01), "Numeric Control 2"=0.0, "TabControl"=enum."Measure"}  # DataQueue
                w854 = T9 {"QueueAction"=enum."TimeOut", "Numeric 1"=0.0, "Numeric 2"=0.0, "Boolean 1"=FALSE, "Boolean 2"=FALSE, "Spin Program"=[], "Spin Prg v07"=[], "Time Stamp"=timestamp(0 s since 1904-01-01), "TabControl"=enum."Measure"}  # Device Queue
                n382 = call-dynamic "Get_WavelengthAxis.vi"("error in (no error)"=w836, "Avantes in"=w838) -> ("error out"=w835:errorcluster, "lambda"=w830:dbl[unit][], "Avantes out"=w837:refnum<class "Avantes.lvclass">)  [unwired: 7 in]
                n383 = property on="Calculate Frames" class="Bool (strict)"() -> ("Value"=w846:bool)  [unwired: 2 in, 2 out]
                n384 = property on="Measure_IntegrationTime" class="DigNum (strict)"() -> ("Value"=w851:dbl[unit])  [unwired: 2 in, 2 out]
                n385 = Unbundle(w835) -> ("status"=w834:bool)  [unwired: 2 out]
                n386 = node(w851) -> (w850:dbl)
                n387 = Bundle By Name(cluster=w854, "QueueAction"=DeviceQueue_Action."Spectrometer_SetIntegrationTime", "Numeric 1"=w850, "Boolean 1"=w846) -> (w848:T9)
                n388 = property on="Frames" class="DigNum (strict)"() -> ("Value"=w845:i32)  [unwired: 2 in, 2 out]
                n389 = property on="Error_Spectromter" class="Bool (strict)"("Value"=w834) -> ()  [unwired: 2 in, 2 out]
                n390 = Enqueue Element(queue=w853, element=w848, error in (no error)=w836) -> (queue out=w849:refnum<queue>, error out=w843:errorcluster)  [unwired: 1 in, 1 out]
                n391 = Bundle By Name(cluster=w848, "QueueAction"=DeviceQueue_Action."Spectrometer_SetFrames", "Numeric 1"=w845) -> (w844:T9)
                n392 = Bundle By Name(cluster=w839, "QueueAction"=DataQueue_Action."Set_Wavelength", "Wavelength"=w830) -> (w840:T6)
                n393 = Enqueue Element(queue=w833, element=w840) -> (queue out=w831:refnum<queue>)  [unwired: 2 in, 2 out]
                n394 = Enqueue Element(queue=w849, element=w844, error in (no error)=w843) -> (queue out=w842:refnum<queue>, error out=w841:errorcluster)  [unwired: 1 in, 1 out]
              }
            }
            n395 = Bundle By Name(cluster=w819, "Abstract_CCD.lvclass"=w814) -> (w813:T5)
          }
          frame "Spectrometer_Close" {
            n396 = property on="Spectromter" class="Bool (strict)"("Value"=FALSE ("Spectromter")) -> ()  [unwired: 2 in, 2 out]
            n397 = Unbundle By Name(w860) -> ("Abstract_CCD.lvclass"=w863:refnum<class "Abstract_CCD.lvclass">)
            n398 = flat-sequence {
              tunnel: [refnum<class "Abstract_CCD.lvclass"> refnum ("Abstract_CCD.lvclass")] -> w857
              tunnel: w856 -> [_]
              frame #0 {
              }
            }
            n399 = call-dynamic "Close.vi"("error in (no error)"=w862, "Abstract_CCD in"=w863) -> ("error out"=w856:errorcluster)  [unwired: 8 in, 1 out]
            n400 = Bundle By Name(cluster=w860, "Abstract_CCD.lvclass"=w857) -> (w859:T5)
          }
          frame "Spectrometer_Measure" {
            w879 = T6 {"QueueAction"=enum."TimeOut", "Data"=[], "Data_Raw"=[], "Data_Dark"=[], "Data_Ref"=[], "Device Information"=[], "Numeric Control"=0.0, "Boolean"=FALSE, "Wavelength"=[], "Time"=[], "Time Stamp"=timestamp(0 s since 1904-01-01), "Numeric Control 2"=0.0, "TabControl"=enum."Measure"}  # DataQueue
            n401 = Unbundle By Name(w874) -> ("Abstract_CCD.lvclass"=w878:refnum<class "Abstract_CCD.lvclass">)
            n402 = Unbundle By Name(w866) -> ("Time Stamp"=w865:timestamp)
            n403 = call-dynamic "Measure.vi"("error in (no error)"=w876, "Abstract_CCD in"=w878) -> ("error out"=w875:errorcluster, "Data Raw"=w871:T12, "Data"=w872:T12, "Darkspec"=w870:T12, "Time"=w869:dbl[])  [unwired: 3 in, 2 out]
            n404 = Bundle By Name(cluster=w879, "QueueAction"=DataQueue_Action."Spectrometer_Measure", "Data"=w872, "Data_Raw"=w871, "Data_Dark"=w870, "Time"=w869, "Time Stamp"=w865) -> (w880:T6)
            n405 = Enqueue Element(queue=w867, element=w880) -> (queue out=w868:refnum<queue>)  [unwired: 2 in, 2 out]
          }
          frame "Spectrometer_MeasureAdvanced" {
            w890 = T6 {"QueueAction"=enum."TimeOut", "Data"=[], "Data_Raw"=[], "Data_Dark"=[], "Data_Ref"=[], "Device Information"=[], "Numeric Control"=0.0, "Boolean"=FALSE, "Wavelength"=[], "Time"=[], "Time Stamp"=timestamp(0 s since 1904-01-01), "Numeric Control 2"=0.0, "TabControl"=enum."Measure"}  # DataQueue
            w904 = T6 {"QueueAction"=enum."TimeOut", "Data"=[], "Data_Raw"=[], "Data_Dark"=[], "Data_Ref"=[], "Device Information"=[], "Numeric Control"=0.0, "Boolean"=FALSE, "Wavelength"=[], "Time"=[], "Time Stamp"=timestamp(0 s since 1904-01-01), "Numeric Control 2"=0.0, "TabControl"=enum."Measure"}  # DataQueue
            n406 = Unbundle By Name(w899) -> ("Abstract_CCD.lvclass"=w903:refnum<class "Abstract_CCD.lvclass">)
            n407 = Unbundle By Name(w893) -> ("Time Stamp"=w892:timestamp)
            n408 = call-dynamic "Measure.vi"("error in (no error)"=w901, "Abstract_CCD in"=w903) -> ("error out"=w900:errorcluster, "Data Raw"=w896:T12, "Data"=w897:T12, "Darkspec"=w895:T12, "Time"=w894:dbl[])  [unwired: 3 in, 2 out]
            n409 = Bundle By Name(cluster=w890, "QueueAction"=DataQueue_Action."Measure_SpectrumAdvanced") -> (w888:T6)
            n410 = Bundle By Name(cluster=w904, "QueueAction"=DataQueue_Action."Spectrometer_Measure", "Data"=w897, "Data_Raw"=w896, "Data_Dark"=w895, "Time"=w894, "Time Stamp"=w892) -> (w885:T6)
            n411 = Enqueue Element(queue=w891, element=w888) -> (queue out=w887:refnum<queue>)  [unwired: 2 in, 2 out]
            n412 = Enqueue Element(queue=w887, element=w885) -> (queue out=w886:refnum<queue>)  [unwired: 2 in, 2 out]
            n413 = Bundle By Name(cluster=w885, "QueueAction"=DataQueue_Action."Stop_Measurement") -> (w883:T6)
            n414 = property on="Action" class="Str"("Value"="Measure Spectra A" ("Action")) -> ()  [unwired: 2 in, 2 out]
            n415 = Enqueue Element(queue=w886, element=w883) -> (queue out=w882:refnum<queue>)  [unwired: 2 in, 2 out]
          }
          frame "Spectrometer_Preview" {
            w918 = T6 {"QueueAction"=enum."TimeOut", "Data"=[], "Data_Raw"=[], "Data_Dark"=[], "Data_Ref"=[], "Device Information"=[], "Numeric Control"=0.0, "Boolean"=FALSE, "Wavelength"=[], "Time"=[], "Time Stamp"=timestamp(0 s since 1904-01-01), "Numeric Control 2"=0.0, "TabControl"=enum."Measure"}  # DataQueue
            n416 = Unbundle By Name(w910) -> ("Abstract_CCD.lvclass"=w908:refnum<class "Abstract_CCD.lvclass">)
            n417 = call-dynamic "Measure.vi"("error in (no error)"=w907, "Abstract_CCD in"=w908) -> ("error out"=w905:errorcluster, "Data Raw"=w915:T12, "Abstract_CCD out"=w906:refnum<class "Abstract_CCD.lvclass">)  [unwired: 3 in, 4 out]
            n418 = property on="Measure_Preview" class="Bool (strict)"(error in=w905) -> ("Value"=w913:bool)  [unwired: 1 in, 2 out]
            n419 = case shown="True" w913 {
              tunnel: [w920 w922] -> w912
              tunnel: w911 -> [w920 w921]
              frame False {
              }
              frame True {
                w924 = T9 {"QueueAction"=enum."TimeOut", "Numeric 1"=0.0, "Numeric 2"=0.0, "Boolean 1"=FALSE, "Boolean 2"=FALSE, "Spin Program"=[], "Spin Prg v07"=[], "Time Stamp"=timestamp(0 s since 1904-01-01), "TabControl"=enum."Measure"}  # Device Queue
                n420 = Bundle By Name(cluster=w924, "QueueAction"=DeviceQueue_Action."Spectrometer_Preview") -> (w923:T9)
                n421 = Enqueue Element(queue=w921, element=w923) -> (queue out=w922:refnum<queue>)  [unwired: 2 in, 2 out]
              }
            }
            n422 = Bundle By Name(cluster=w918, "Data_Raw"=w915, "QueueAction"=DataQueue_Action."Spectrometer_Preview") -> (w919:T6)
            n423 = Enqueue Element(queue=w917, element=w919) -> (queue out=w916:refnum<queue>)  [unwired: 2 in, 2 out]
            n424 = Bundle By Name(cluster=w910, "Abstract_CCD.lvclass"=w906) -> (w909:T5)
          }
          frame "Spectrometer_StartMeasurement" {
            n425 = Unbundle By Name(w928) -> ("Abstract_CCD.lvclass"=w932:refnum<class "Abstract_CCD.lvclass">)
            n426 = call-dynamic "StartMeasure.vi"("error in (no error)"=w933, "Frames"=-1, "Abstract_CCD in"=w932) -> ("error out"=w931:errorcluster, "Abstract_CCD out"=w927:refnum<class "Abstract_CCD.lvclass">)  [unwired: 7 in]
            n427 = Bundle By Name(cluster=w928, "Abstract_CCD.lvclass"=w927) -> (w926:T5)
          }
          frame "Spectrometer_StopMeasurement" {
            n428 = Unbundle By Name(w940) -> ("Abstract_CCD.lvclass"=w942:refnum<class "Abstract_CCD.lvclass">)
            n429 = call-dynamic "StopMeasurement.vi"("error in (no error)"=w941, "Abstract_CCD in"=w942) -> ("error out"=w938:errorcluster, "Abstract_CCD out"=w939:refnum<class "Abstract_CCD.lvclass">)  [unwired: 8 in]
            n430 = Bundle By Name(cluster=w940, "Abstract_CCD.lvclass"=w939) -> (w935:T5)
          }
          frame "Spectrometer_GetData" {
            w952 = T6 {"QueueAction"=enum."TimeOut", "Data"=[], "Data_Raw"=[], "Data_Dark"=[], "Data_Ref"=[], "Device Information"=[], "Numeric Control"=0.0, "Boolean"=FALSE, "Wavelength"=[], "Time"=[], "Time Stamp"=timestamp(0 s since 1904-01-01), "Numeric Control 2"=0.0, "TabControl"=enum."Measure"}  # DataQueue
            n431 = Unbundle By Name(w949) -> ("Abstract_CCD.lvclass"=w954:refnum<class "Abstract_CCD.lvclass">)
            n432 = Unbundle By Name(w955) -> ("Numeric 1"=w946:dbl)
            n433 = call-dynamic "Measure_GetData.vi"("error in (no error)"=w953, "SpectraCount"=w946, "Abstract_CCD in"=w954) -> ("error out"=w943:errorcluster, "Data_Raw"=w945:T12, "Time"=w944:dbl[])  [unwired: 5 in, 1 out]
            n434 = Bundle By Name(cluster=w952, "QueueAction"=DataQueue_Action."Spectrometer_Measure", "Data_Raw"=w945, "Time"=w944) -> (w951:T6)
            n435 = Enqueue Element(queue=w948, element=w951) -> (queue out=w947:refnum<queue>)  [unwired: 2 in, 2 out]
          }
          frame "Spectrometer_SetIntegrationTime" {
            n436 = Unbundle By Name(w964) -> ("Numeric 1"=w966:dbl)
            n437 = Unbundle By Name(w960) -> ("Abstract_CCD.lvclass"=w968:refnum<class "Abstract_CCD.lvclass">)
            n438 = Unbundle By Name(w964) -> ("Boolean 1"=w963:bool)
            n439 = node(w966) -> (w965:dbl[unit])
            n440 = call-dynamic "Set_ExposureTime.vi"("error in (no error)"=w967, "Exposure Time"=w965, "Abstract_CCD in"=w968) -> ("error out"=w971:errorcluster, "Abstract_CCD out"=w970:refnum<class "Abstract_CCD.lvclass">)  [unwired: 7 in]
            n441 = call-dynamic "Get_FrameRate.vi"("error in (no error)"=w971, "Abstract_CCD in"=w970) -> ("error out"=w961:errorcluster, "Frame Rate"=w962:dbl[unit], "Abstract_CCD out"=w959:refnum<class "Abstract_CCD.lvclass">)  [unwired: 7 in]
            "Measure_FrameRate" <- w962
            n442 = Bundle By Name(cluster=w960, "Abstract_CCD.lvclass"=w959) -> (w958:T5)
            n443 = case shown="True" w963 {
              tunnel: w962 -> [_ w975]
              frame False {
              }
              frame True {
                n444 = property on="Program Spin Coater" class="Arr (strict)"() -> ("Value"=w972:T2)  [unwired: 2 in, 2 out]
                n445 = property on="Seconds to Spin" class="DigNum (strict)"() -> ("Value"=w977:dbl[unit])  [unwired: 2 in, 2 out]
                n446 = property on="Seconds after Spin" class="DigNum (strict)"() -> ("Value"=w976:dbl[unit])  [unwired: 2 in, 2 out]
                n447 = call "CalculateFrames_v02.vi"("Program Spin Coater"=w972, "Seconds End"=w976, "Seconds Start"=w977, "Frame Rate"=w975) -> ("Time"=w974:dbl, "Frames"=w973:i32)  [unwired: 6 in]
                n448 = property on="Overall Time" class="DigNum (strict)"("Value"=w974) -> ()  [unwired: 2 in, 2 out]
                n449 = property on="Frames" class="DigNum (strict)"("Value"=w973) -> ()  [unwired: 2 in, 2 out]
              }
            }
          }
          frame "Spectrometer_SetFrames" {
            n450 = Unbundle By Name(w979) -> ("Abstract_CCD.lvclass"=w984:refnum<class "Abstract_CCD.lvclass">)
            n451 = Unbundle By Name(w987) -> ("Numeric 1"=w981:dbl)
            n452 = call-dynamic "Set_Frames.vi"("error in (no error)"=w983, "Frames"=w981, "Abstract_CCD in"=w984) -> ("error out"=w982:errorcluster, "Abstract_CCD out"=w978:refnum<class "Abstract_CCD.lvclass">)  [unwired: 7 in]
            n453 = Bundle By Name(cluster=w979, "Abstract_CCD.lvclass"=w978) -> (w980:T5)
          }
          frame "Spectrometer_SetDarkspec" {
            w1000 = T6 {"QueueAction"=enum."TimeOut", "Data"=[], "Data_Raw"=[], "Data_Dark"=[], "Data_Ref"=[], "Device Information"=[], "Numeric Control"=0.0, "Boolean"=FALSE, "Wavelength"=[], "Time"=[], "Time Stamp"=timestamp(0 s since 1904-01-01), "Numeric Control 2"=0.0, "TabControl"=enum."Measure"}  # DataQueue
            n454 = Unbundle By Name(w995) -> ("Abstract_CCD.lvclass"=w993:refnum<class "Abstract_CCD.lvclass">)
            n455 = call-dynamic "Measure.vi"("error in (no error)"=w992, "Abstract_CCD in"=w993) -> ("error out"=w990:errorcluster, "Data Raw"=w997:T12, "Abstract_CCD out"=w991:refnum<class "Abstract_CCD.lvclass">)  [unwired: 3 in, 4 out]
            n456 = Bundle By Name(cluster=w1000, "QueueAction"=DataQueue_Action."Set_Dark", "Data_Dark"=w997) -> (w1001:T6)
            n457 = Enqueue Element(queue=w999, element=w1001) -> (queue out=w996:refnum<queue>)  [unwired: 2 in, 2 out]
            n458 = Bundle By Name(cluster=w995, "Abstract_CCD.lvclass"=w991) -> (w994:T5)
            n459 = property on="Record_Darkspec" class="Bool (strict)"(error in=w990, "Value"=FALSE ("Record_Darkspec")) -> (error out=w989:errorcluster)  [unwired: 1 in, 1 out]
          }
          frame "Spectrometer_SetReference" {
            w1015 = T6 {"QueueAction"=enum."TimeOut", "Data"=[], "Data_Raw"=[], "Data_Dark"=[], "Data_Ref"=[], "Device Information"=[], "Numeric Control"=0.0, "Boolean"=FALSE, "Wavelength"=[], "Time"=[], "Time Stamp"=timestamp(0 s since 1904-01-01), "Numeric Control 2"=0.0, "TabControl"=enum."Measure"}  # DataQueue
            n460 = Unbundle By Name(w1010) -> ("Abstract_CCD.lvclass"=w1007:refnum<class "Abstract_CCD.lvclass">)
            n461 = call-dynamic "Measure.vi"("error in (no error)"=w1008, "Abstract_CCD in"=w1007) -> ("error out"=w1005:errorcluster, "Data Raw"=w1012:T12, "Abstract_CCD out"=w1006:refnum<class "Abstract_CCD.lvclass">)  [unwired: 3 in, 4 out]
            n462 = Bundle By Name(cluster=w1015, "QueueAction"=DataQueue_Action."Set_Ref", "Data_Ref"=w1012) -> (w1016:T6)
            n463 = Enqueue Element(queue=w1014, element=w1016) -> (queue out=w1011:refnum<queue>)  [unwired: 2 in, 2 out]
            n464 = Bundle By Name(cluster=w1010, "Abstract_CCD.lvclass"=w1006) -> (w1009:T5)
            n465 = property on="Record RefSpec" class="Bool (strict)"(error in=w1005, "Value"=FALSE ("Record RefSpec")) -> (error out=w1004:errorcluster)  [unwired: 1 in, 1 out]
          }
          frame "Spectrometer_SetTriggerMode" {
            n466 = Unbundle By Name(w1021) -> ("Abstract_CCD.lvclass"=w1026:refnum<class "Abstract_CCD.lvclass">)
            n467 = Unbundle By Name(w1025) -> ("Numeric 1"=w1023:dbl)
            n468 = call-dynamic "Set_TriggerMode.vi"("error in (no error)"=w1024, "Trigger Mode"=w1023, "Abstract_CCD in"=w1026) -> ("error out"=w1022:errorcluster, "Abstract_CCD out"=w1020:refnum<class "Abstract_CCD.lvclass">)  [unwired: 7 in]
            n469 = Bundle By Name(cluster=w1021, "Abstract_CCD.lvclass"=w1020) -> (w1019:T5)
          }
          frame "Spectrometer_DeviceInformation" {
            w1034 = T6 {"QueueAction"=enum."TimeOut", "Data"=[], "Data_Raw"=[], "Data_Dark"=[], "Data_Ref"=[], "Device Information"=[], "Numeric Control"=0.0, "Boolean"=FALSE, "Wavelength"=[], "Time"=[], "Time Stamp"=timestamp(0 s since 1904-01-01), "Numeric Control 2"=0.0, "TabControl"=enum."Measure"}  # DataQueue
            n470 = Unbundle By Name(w1028) -> ("Abstract_CCD.lvclass"=w1036:refnum<class "Abstract_CCD.lvclass">)
            n471 = call-dynamic "Get_DeviceInformation.vi"("error in (no error)"=w1035, "Abstract_CCD in"=w1036) -> ("error out"=w1030:errorcluster, "Array"=w1037:string[])  [unwired: 7 in, 1 out]
            n472 = Bundle By Name(cluster=w1034, "QueueAction"=DataQueue_Action."Transfer_Settings", "Device Information"=w1037) -> (w1032:T6)
            n473 = Enqueue Element(queue=w1033, element=w1032, error in (no error)=w1030) -> (queue out=w1031:refnum<queue>, error out=w1029:errorcluster)  [unwired: 1 in, 1 out]
          }
          frame "Arduino_Init" {
            n474 = Unbundle By Name(w1048) -> ("SpinCoater.lvclass"=w1047:refnum<class "SpinCoater.lvclass">)
            n475 = call-dynamic "Init.vi"("error in (no error)"=w1046, "Variant"="Port Arduino", "SpinCoater in"=w1047) -> ("error out"=w1043:errorcluster, "SpinCoater out"=w1044:refnum<class "SpinCoater.lvclass">)  [unwired: 7 in]
            n476 = call-dynamic "IsInit.vi"("error in (no error)"=w1043, "SpinCoater in"=w1044) -> ("error out"=w1040:errorcluster, "Init"=w1041:bool, "SpinCoater out"=w1042:refnum<class "SpinCoater.lvclass">)  [unwired: 7 in]
            n477 = property on="Arduino" class="Bool (strict)"("Value"=w1041) -> ()  [unwired: 2 in, 2 out]
            n478 = case shown="True" w1041 {
              tunnel: w1051 -> [w1055 w1064]
              tunnel: [w1055 w1058] -> w1050
              tunnel: [w1054 w1057] -> w1049
              tunnel: w1040 -> [w1054 w1061]
              frame False {
              }
              frame True {
                w1065 = T9 {"QueueAction"=enum."TimeOut", "Numeric 1"=0.0, "Numeric 2"=0.0, "Boolean 1"=FALSE, "Boolean 2"=FALSE, "Spin Program"=[], "Spin Prg v07"=[], "Time Stamp"=timestamp(0 s since 1904-01-01), "TabControl"=enum."Measure"}  # Device Queue
                n479 = property on="Program Spin Coater" class="Arr (strict)"() -> ("Value"=w1056:T2)  [unwired: 2 in, 2 out]
                n480 = property on="Seconds to Spin" class="DigNum (strict)"() -> ("Value"=w1060:dbl[unit])  [unwired: 2 in, 2 out]
                n481 = node(w1060) -> (w1059:dbl)
                n482 = Bundle By Name(cluster=w1065, "QueueAction"=DeviceQueue_Action."Arduino_LoadProgram", "Spin Prg v07"=w1056, "Numeric 1"=w1059) -> (w1063:T9)
                n483 = Enqueue Element(queue=w1064, element=w1063, error in (no error)=w1061) -> (queue out=w1058:refnum<queue>, error out=w1057:errorcluster)  [unwired: 1 in, 1 out]
              }
            }
            n484 = Bundle By Name(cluster=w1048, "SpinCoater.lvclass"=w1042) -> (w1052:T5)
          }
          frame "Arduino_Close" {
            n485 = Unbundle By Name(w1068) -> ("SpinCoater.lvclass"=w1076:refnum<class "SpinCoater.lvclass">)
            n486 = property on="Arduino" class="Bool (strict)"() -> (error out=w1070:errorcluster, "Value"=w1069:bool)  [unwired: 2 in, 1 out]
            n487 = property on="Arduino" class="Bool (strict)"(error in=w1070, "Value"=FALSE ("Arduino")) -> ()  [unwired: 1 in, 2 out]
            n488 = case shown="False" w1069 {
              tunnel: w1076 -> [w1077 w1082]
              tunnel: w1075 -> [w1078 w1081]
              tunnel: [w1078 w1080] -> w1074
              tunnel: [w1077 w1079] -> w1067
              frame False {
              }
              frame True {
                n489 = call-dynamic "Close.vi"("error in (no error)"=w1081, "SpinCoater in"=w1082) -> ("error out"=w1080:errorcluster, "SpinCoater out"=w1079:refnum<class "SpinCoater.lvclass">)  [unwired: 8 in]
              }
            }
            n490 = Bundle By Name(cluster=w1068, "SpinCoater.lvclass"=w1067) -> (w1066:T5)
          }
          frame "Arduino_LoadProgram" {
            n491 = Unbundle By Name(w1092) -> ("Spin Prg v07"=w1083:T2, "Numeric 1"=w1091:dbl)
            n492 = Unbundle By Name(w1087) -> ("SpinCoater.lvclass"=w1090:refnum<class "SpinCoater.lvclass">)
            n493 = node(w1091) -> (w1089:dbl[unit])
            n494 = call-dynamic "Program_Load_v02.vi"("error in (no error)"=w1088, "Time Start"=w1089, "Program Spin Coater"=w1083, "SpinCoater in"=w1090) -> ("error out"=w1085:errorcluster, "SpinCoater out"=w1086:refnum<class "SpinCoater.lvclass">)  [unwired: 6 in]
            n495 = Bundle By Name(cluster=w1087, "SpinCoater.lvclass"=w1086) -> (w1084:T5)
          }
          frame "Arduino_StartProgram" {
            n496 = Unbundle By Name(w1100) -> ("SpinCoater.lvclass"=w1097:refnum<class "SpinCoater.lvclass">)
            n497 = call-dynamic "Program_Run.vi"("error in (no error)"=w1096, "SpinCoater in"=w1097) -> ("error out"=w1095:errorcluster)  [unwired: 8 in, 1 out]
            n498 = property on="Action" class="Str"("Value"="Measuring" ("Action")) -> ()  [unwired: 2 in, 2 out]
          }
          frame "Arduino_SetSpeed" {
            n499 = Unbundle By Name(w1109) -> ("SpinCoater.lvclass"=w1105:refnum<class "SpinCoater.lvclass">)
            n500 = Unbundle By Name(w1108) -> ("Numeric 1"=w1107:dbl)
            n501 = To Unsigned Long Integer(number=w1107) -> (unsigned 32bit integer=w1103:u32)
            n502 = call-dynamic "Debug_SetSpeed.vi"("error in (no error)"=w1104, "Speed"=w1103, "SpinCoater in"=w1105) -> ("error out"=w1102:errorcluster)  [unwired: 7 in, 1 out]
          }
          frame "Arduino_SetMillis" {
            n503 = Unbundle By Name(w1115) -> ("SpinCoater.lvclass"=w1114:refnum<class "SpinCoater.lvclass">)
            n504 = Unbundle By Name(w1117) -> ("Numeric 1"=w1119:dbl)
            n505 = To Unsigned Long Integer(number=w1119) -> (unsigned 32bit integer=w1111:u32)
            n506 = call-dynamic "Debug_SetMillis.vi"("error in (no error)"=w1113, "Milliseconds"=w1111, "SpinCoater in"=w1114) -> ("error out"=w1112:errorcluster)  [unwired: 7 in, 1 out]
          }
          frame "Arduino_StopSpin" {
            n507 = Unbundle By Name(w1123) -> ("SpinCoater.lvclass"=w1122:refnum<class "SpinCoater.lvclass">)
            n508 = call-dynamic "Stop_Spin.vi"("error in (no error)"=w1121, "SpinCoater in"=w1122) -> ("error out"=w1120:errorcluster)  [unwired: 8 in, 1 out]
          }
          frame "Measure_Stop" {
            w1132 = T6 {"QueueAction"=enum."TimeOut", "Data"=[], "Data_Raw"=[], "Data_Dark"=[], "Data_Ref"=[], "Device Information"=[], "Numeric Control"=0.0, "Boolean"=FALSE, "Wavelength"=[], "Time"=[], "Time Stamp"=timestamp(0 s since 1904-01-01), "Numeric Control 2"=0.0, "TabControl"=enum."Measure"}  # DataQueue
            n509 = Bundle By Name(cluster=w1132, "QueueAction"=DataQueue_Action."Stop_Measurement") -> (w1133:T6)
            n510 = Enqueue Element(queue=w1130, element=w1133, error in (no error)=w1127) -> (queue out=w1129:refnum<queue>, error out=w1126:errorcluster)  [unwired: 1 in, 1 out]
          }
          frame "Measure_InSitu" {
            w1174 = T9 {"QueueAction"=enum."TimeOut", "Numeric 1"=0.0, "Numeric 2"=0.0, "Boolean 1"=FALSE, "Boolean 2"=FALSE, "Spin Program"=[], "Spin Prg v07"=[], "Time Stamp"=timestamp(0 s since 1904-01-01), "TabControl"=enum."Measure"}  # Device Queue
            w1181 = T9 {"QueueAction"=enum."TimeOut", "Numeric 1"=0.0, "Numeric 2"=0.0, "Boolean 1"=FALSE, "Boolean 2"=FALSE, "Spin Program"=[], "Spin Prg v07"=[], "Time Stamp"=timestamp(0 s since 1904-01-01), "TabControl"=enum."Measure"}  # Device Queue
            n511 = Bundle By Name(cluster=w1181, "QueueAction"=DeviceQueue_Action."Spectrometer_SetTriggerMode", "Numeric 1"=1.0) -> (w1179:T9)
            n512 = Bundle By Name(cluster=w1174, "QueueAction"=DeviceQueue_Action."Spectrometer_DeviceInformation") -> (w1171:T9)
            n513 = Bundle By Name(cluster=w1171, "QueueAction"=DeviceQueue_Action."Spectrometer_StartMeasurement") -> (w1167:T9)
            n514 = Enqueue Element(queue=w1180, element=w1179, error in (no error)=w1136) -> (queue out=w1176:refnum<queue>, error out=w1177:errorcluster)  [unwired: 1 in, 1 out]
            n515 = property on="Frames" class="DigNum (strict)"() -> ("Value"=w1137:i32)  [unwired: 2 in, 2 out]
            n516 = Bundle By Name(cluster=w1167, "QueueAction"=DeviceQueue_Action."Arduino_StartProgram") -> (w1162:T9)
            n517 = Enqueue Element(queue=w1176, element=w1171, error in (no error)=w1177) -> (queue out=w1173:refnum<queue>, error out=w1172:errorcluster)  [unwired: 1 in, 1 out]
            n518 = Bundle By Name(cluster=w1162, "QueueAction"=DeviceQueue_Action."Spectrometer_GetData", "Numeric 1"="Dividider Get Spectra") -> (w1157:T9)
            n519 = Divide(x=w1137, y="Dividider Get Spectra") -> (x/y=w1169:dbl)
            n520 = Round Toward +Infinity(x=w1169) -> (ceil(x): smallest int >= x=w1168:dbl)
            n521 = Enqueue Element(queue=w1173, element=w1167, error in (no error)=w1172) -> (queue out=w1166:refnum<queue>, error out=w1165:errorcluster)  [unwired: 1 in, 1 out]
            n522 = Enqueue Element(queue=w1166, element=w1162, error in (no error)=w1165) -> (queue out=w1163:refnum<queue>, error out=w1160:errorcluster)  [unwired: 1 in, 1 out]
            n523 = for {
              N: w1168 -> [_]
              shift-right: [w1184] -> w1159
              shift-left: w1163 -> [w1188]
              tunnel: w1157 -> [w1185]
              shift-right: [w1186] -> w1158
              shift-left: w1160 -> [w1187]
              n524 = Enqueue Element(queue=w1188, element=w1185, error in (no error)=w1187) -> (queue out=w1184:refnum<queue>, error out=w1186:errorcluster)  [unwired: 1 in, 1 out]
            }
            n525 = Bundle By Name(cluster=w1157, "QueueAction"=DeviceQueue_Action."Spectrometer_StopMeasurement") -> (w1153:T9)
            n526 = property on="Measure_FramesSpectrometer" class="DigNum (strict)"() -> ("Value"=w1139:dbl)  [unwired: 2 in, 2 out]
            n527 = Bundle By Name(cluster=w1153, "QueueAction"=DeviceQueue_Action."Measure_Stop") -> (w1146:T9)
            n528 = Enqueue Element(queue=w1159, element=w1153, error in (no error)=w1158) -> (queue out=w1154:refnum<queue>, error out=w1155:errorcluster)  [unwired: 1 in, 1 out]
            n529 = Bundle By Name(cluster=w1146, "QueueAction"=DeviceQueue_Action."Spectrometer_SetTriggerMode", "Numeric 1"=0.0) -> (w1141:T9)
            n530 = Enqueue Element(queue=w1154, element=w1146, error in (no error)=w1155) -> (queue out=w1149:refnum<queue>, error out=w1150:errorcluster)  [unwired: 1 in, 1 out]
            n531 = Bundle By Name(cluster=w1141, "QueueAction"=DeviceQueue_Action."Spectrometer_SetFrames", "Numeric 1"=w1139) -> (w1138:T9)
            n532 = Enqueue Element(queue=w1149, element=w1141, error in (no error)=w1150) -> (queue out=w1148:refnum<queue>, error out=w1147:errorcluster)  [unwired: 1 in, 1 out]
            n533 = Enqueue Element(queue=w1148, element=w1138, error in (no error)=w1147) -> (queue out=w1142:refnum<queue>, error out=w1143:errorcluster)  [unwired: 1 in, 1 out]
          }
          frame "Measure_InSituAdvanced" {
            w1271 = T9 {"QueueAction"=enum."TimeOut", "Numeric 1"=0.0, "Numeric 2"=0.0, "Boolean 1"=FALSE, "Boolean 2"=FALSE, "Spin Program"=[], "Spin Prg v07"=[], "Time Stamp"=timestamp(0 s since 1904-01-01), "TabControl"=enum."Measure"}  # Device Queue
            n534 = property on="Dividider Get Spectra" class="DigNum (strict)"() -> ("Value"=w1230:u32)  [unwired: 2 in, 2 out]
            n535 = Bundle By Name(cluster=w1271, "QueueAction"=DeviceQueue_Action."Spectrometer_SetTriggerMode", "Numeric 1"=1.0) -> (w1226:T9)
            n536 = Bundle By Name(cluster=w1226, "QueueAction"=DeviceQueue_Action."Spectrometer_DeviceInformation") -> (w1263:T9)
            n537 = Bundle By Name(cluster=w1263, "QueueAction"=DeviceQueue_Action."Spectrometer_StartMeasurement") -> (w1259:T9)
            n538 = Enqueue Element(queue=w1270, element=w1226, error in (no error)=w1231) -> (queue out=w1267:refnum<queue>, error out=w1268:errorcluster)  [unwired: 1 in, 1 out]
            n539 = Bundle By Name(cluster=w1259, "QueueAction"=DeviceQueue_Action."Arduino_StartProgram") -> (w1254:T9)
            n540 = property on="Frames" class="DigNum (strict)"() -> ("Value"=w1232:i32)  [unwired: 2 in, 2 out]
            n541 = Unbundle By Name(w1213) -> ("Time Stamp"=w1212:timestamp)
            n542 = Enqueue Element(queue=w1267, element=w1263, error in (no error)=w1268) -> (queue out=w1265:refnum<queue>, error out=w1264:errorcluster)  [unwired: 1 in, 1 out]
            n543 = Bundle By Name(cluster=w1254, "QueueAction"=DeviceQueue_Action."Spectrometer_GetData", "Numeric 1"=w1230) -> (w1249:T9)
            n544 = Divide(x=w1232, y=w1230) -> (x/y=w1261:dbl)
            n545 = Round Toward +Infinity(x=w1261) -> (ceil(x): smallest int >= x=w1260:dbl)
            n546 = Enqueue Element(queue=w1265, element=w1259, error in (no error)=w1264) -> (queue out=w1258:refnum<queue>, error out=w1257:errorcluster)  [unwired: 1 in, 1 out]
            n547 = Enqueue Element(queue=w1258, element=w1254, error in (no error)=w1257) -> (queue out=w1255:refnum<queue>, error out=w1252:errorcluster)  [unwired: 1 in, 1 out]
            n548 = Bundle By Name(cluster=w1249, "QueueAction"=DeviceQueue_Action."Spectrometer_StopMeasurement") -> (w1245:T9)
            n549 = for {
              N: w1260 -> [_]
              shift-right: [w1321] -> w1251
              shift-left: w1255 -> [w1325]
              tunnel: w1249 -> [w1322]
              shift-right: [w1323] -> w1250
              shift-left: w1252 -> [w1324]
              n550 = Enqueue Element(queue=w1325, element=w1322, error in (no error)=w1324) -> (queue out=w1321:refnum<queue>, error out=w1323:errorcluster)  [unwired: 1 in, 1 out]
            }
            n551 = property on="Measure_FramesSpectrometer" class="DigNum (strict)"() -> ("Value"=w1233:dbl)  [unwired: 2 in, 2 out]
            n552 = property on="periodic time" class="DigNum (strict)"() -> ("Value"=w1225:dbl[unit])  [unwired: 2 in, 2 out]
            n553 = Bundle By Name(cluster=w1245, "QueueAction"=DeviceQueue_Action."Measure_Stop") -> (w1238:T9)
            n554 = property on="Duration after" class="DigNum (strict)"() -> ("Value"=w1224:dbl[unit])  [unwired: 2 in, 2 out]
            n555 = node(w1225) -> (w1192:dbl)
            n556 = property on="periodic time" class="DigNum (strict)"() -> ("Value"=w1223:dbl[unit])  [unwired: 2 in, 2 out]
            n557 = Bundle By Name(cluster=w1238, "QueueAction"=DeviceQueue_Action."Spectrometer_SetTriggerMode", "Numeric 1"=0.0) -> (w1235:T9)
            n558 = Enqueue Element(queue=w1251, element=w1245, error in (no error)=w1250) -> (queue out=w1246:refnum<queue>, error out=w1247:errorcluster)  [unwired: 1 in, 1 out]
            n559 = node(w1224) -> (w1218:dbl)
            n560 = Bundle By Name(cluster=w1235, "QueueAction"=DeviceQueue_Action."Spectrometer_SetFrames", "Numeric 1"=w1233) -> (w1215:T9)
            n561 = Enqueue Element(queue=w1246, element=w1238, error in (no error)=w1247) -> (queue out=w1241:refnum<queue>, error out=w1242:errorcluster)  [unwired: 1 in, 1 out]
            n562 = node(w1223) -> (w1217:dbl)
            n563 = Bundle By Name(cluster=w1215, "QueueAction"=DeviceQueue_Action."Wait", "Numeric 1"=w1192) -> (w1194:T9)
            n564 = Enqueue Element(queue=w1241, element=w1235, error in (no error)=w1242) -> (queue out=w1240:refnum<queue>, error out=w1239:errorcluster)  [unwired: 1 in, 1 out]
            n565 = Not Equal To 0?(x=w1217) -> (x != 0?=w1221:bool)
            n566 = Not Equal To 0?(x=w1218) -> (x != 0?=w1222:bool)
            n567 = Divide(x=w1218, y=w1217) -> (x/y=w1219:dbl)
            n568 = Bundle By Name(cluster=w1194, "QueueAction"=DeviceQueue_Action."Spectrometer_MeasureAdvanced", "Time Stamp"=w1212) -> (w1193:T9)
            n569 = And(x=w1222, y=w1221) -> (x .and. y?=w1220:bool)
            n570 = Round Toward +Infinity(x=w1219) -> (ceil(x): smallest int >= x=w1216:dbl)
            n571 = Enqueue Element(queue=w1240, element=w1215, error in (no error)=w1239) -> (queue out=w1229:refnum<queue>, error out=w1228:errorcluster)  [unwired: 1 in, 1 out]
            n572 = Bundle By Name(cluster=w1193, "QueueAction"=DeviceQueue_Action."Arduino_SetSpeed", "Numeric 1"=1500.0) -> (w1207:T9)
            n573 = Bundle By Name(cluster=w1207, "Numeric 1"=0.0) -> (w1198:T9)
            n574 = property on="Measure_FrameRate" class="DigNum (strict)"() -> ("Value"=w1204:dbl[unit])  [unwired: 2 in, 2 out]
            n575 = property on="Measure_FramesSpectrometer" class="DigNum (strict)"() -> ("Value"=w1203:dbl)  [unwired: 2 in, 2 out]
            n576 = Divide(x=w1203, y=w1204) -> (x/y=w1205:dbl[unit])
            n577 = Bundle By Name(cluster=w1194, "Numeric 1"=1.0) -> (w1200:T9)
            n578 = node(w1205) -> (w1191:dbl)
            n579 = Subtract(x=w1192, y=w1191) -> (x-y=w1190:dbl)
            n580 = Bundle By Name(cluster=w1194, "Numeric 1"=w1190) -> (w1189:T9)
            n581 = Round Toward +Infinity(x=w1191) -> (ceil(x): smallest int >= x=w1206:dbl)
            n582 = Add(x=w1206, y=2.0) -> (x+y=w1201:dbl)
            n583 = Bundle By Name(cluster=w1200, "Numeric 1"=w1201) -> (w1199:T9)
            n584 = case shown="True" w1220 {
              tunnel: w1229 -> [w1275 w1277]
              tunnel: w1228 -> [w1274 w1280]
              tunnel: w1216 -> [_ w1293]
              tunnel: w1193 -> [_ w1292]
              tunnel: w1189 -> [_ w1288]
              tunnel: w1207 -> [_ w1287]
              tunnel: w1200 -> [_ w1286]
              tunnel: w1193 -> [_ w1285]
              tunnel: w1199 -> [_ w1284]
              tunnel: w1198 -> [_ w1283]
              tunnel: [w1274 w1282] -> w1197
              tunnel: [w1275 w1281] -> w1196
              tunnel: w1194 -> [_ w1276]
              frame False {
              }
              frame True {
                n585 = Enqueue Element(queue=w1277, element=w1276, error in (no error)=w1280) -> (queue out=w1278:refnum<queue>, error out=w1279:errorcluster)  [unwired: 1 in, 1 out]
                n586 = for {
                  N: w1293 -> [_]
                  shift-right: [w1314] -> w1290
                  shift-left: w1278 -> [w1320]
                  shift-right: [w1313] -> w1289
                  shift-left: w1279 -> [w1319]
                  tunnel: w1292 -> [w1318]
                  tunnel: w1288 -> [w1315]
                  n587 = Enqueue Element(queue=w1320, element=w1318, error in (no error)=w1319) -> (queue out=w1316:refnum<queue>, error out=w1317:errorcluster)  [unwired: 1 in, 1 out]
                  n588 = Enqueue Element(queue=w1316, element=w1315, error in (no error)=w1317) -> (queue out=w1314:refnum<queue>, error out=w1313:errorcluster)  [unwired: 1 in, 1 out]
                }
                n589 = case shown="True" "Spin at end" {
                  tunnel: w1290 -> [w1295 w1312]
                  tunnel: w1289 -> [w1294 w1311]
                  tunnel: w1287 -> [_ w1306]
                  tunnel: w1286 -> [_ w1305]
                  tunnel: w1285 -> [_ w1304]
                  tunnel: w1284 -> [_ w1299]
                  tunnel: w1283 -> [_ w1298]
                  tunnel: [w1294 w1297] -> w1282
                  tunnel: [w1295 w1296] -> w1281
                  frame False {
                  }
                  frame True {
                    n590 = Enqueue Element(queue=w1312, element=w1306, error in (no error)=w1311) -> (queue out=w1310:refnum<queue>, error out=w1309:errorcluster)  [unwired: 1 in, 1 out]
                    n591 = Enqueue Element(queue=w1310, element=w1305, error in (no error)=w1309) -> (queue out=w1308:refnum<queue>, error out=w1307:errorcluster)  [unwired: 1 in, 1 out]
                    n592 = Enqueue Element(queue=w1308, element=w1304, error in (no error)=w1307) -> (queue out=w1303:refnum<queue>, error out=w1302:errorcluster)  [unwired: 1 in, 1 out]
                    n593 = Enqueue Element(queue=w1303, element=w1299, error in (no error)=w1302) -> (queue out=w1300:refnum<queue>, error out=w1301:errorcluster)  [unwired: 1 in, 1 out]
                    n594 = Enqueue Element(queue=w1300, element=w1298, error in (no error)=w1301) -> (queue out=w1296:refnum<queue>, error out=w1297:errorcluster)  [unwired: 1 in, 1 out]
                  }
                }
              }
            }
            "Nr After Spin" <- u16 0 ("Nr After Spin")
          }
          frame "Measure_Spectrum" {
            w1340 = T9 {"QueueAction"=enum."TimeOut", "Numeric 1"=0.0, "Numeric 2"=0.0, "Boolean 1"=FALSE, "Boolean 2"=FALSE, "Spin Program"=[], "Spin Prg v07"=[], "Time Stamp"=timestamp(0 s since 1904-01-01), "TabControl"=enum."Measure"}  # Device Queue
            n595 = Unbundle By Name(w1327) -> ("Time Stamp"=w1326:timestamp)
            n596 = Bundle By Name(cluster=w1340, "QueueAction"=DeviceQueue_Action."Spectrometer_Measure", "Time Stamp"=w1326) -> (w1332:T9)
            n597 = Bundle By Name(cluster=w1332, "QueueAction"=DeviceQueue_Action."Measure_Stop") -> (w1330:T9)
            n598 = Enqueue Element(queue=w1338, element=w1332, error in (no error)=w1337) -> (queue out=w1333:refnum<queue>, error out=w1334:errorcluster)  [unwired: 1 in, 1 out]
            n599 = Enqueue Element(queue=w1333, element=w1330, error in (no error)=w1334) -> (queue out=w1329:refnum<queue>, error out=w1328:errorcluster)  [unwired: 1 in, 1 out]
          }
        }
      }
      frame Error {
        w1345 = T17 4 items=["no dialog", "OK message", "continue or stop message", "OK message + warnings", "continue/stop + warnings"] ("type of dialog (OK msg:1)")
        n600 = call <vilib>:"General Error Handler.vi"("type of dialog (OK msg:1)"=w1345, "error in (no error)"=w1346) -> ("error out"=w1344:errorcluster)  [unwired: 9 in, 4 out]
        n601 = call <vilib>:"Clear Errors.vi"("error in (no error)"=w1344) -> ("error out"=w1343:errorcluster)  [unwired: 5 in, 1 out]
      }
    }
  }
  n602 = disable-structure shown="Disabled" {
    frame Disabled {
      w1349 = T9 {"QueueAction"=enum."TimeOut", "Numeric 1"=0.0, "Numeric 2"=0.0, "Boolean 1"=FALSE, "Boolean 2"=FALSE, "Spin Program"=[], "Spin Prg v07"=[], "Time Stamp"=timestamp(0 s since 1904-01-01), "TabControl"=enum."Measure"}  # Device Queue
      n603 = Bundle By Name(cluster=w1349, "QueueAction"=DeviceQueue_Action."Arduino_SetSpeed") -> (w1348:T9)  [unwired: 1 in]
      n604 = Enqueue Element(element=w1348) -> ()  [unwired: 3 in, 3 out]
    }
    frame Enabled {
    }
  }
  n605 = Release Queue(queue=w9) -> ()  [unwired: 2 in, 3 out]
  n606 = Release Queue(queue=w10) -> ()  [unwired: 2 in, 3 out]
